vi "Main-GUI-v2.vi"() -> ()   [LabVIEW 2021]
uses:
  Controls/Command_cluster.ctl
  Controls/Command_Enum.ctl
  Controls/AR-msg-variables.ctl
  Controls/AR-com-ports.ctl
  Controls/AR-instrument-refs.ctl
  C:/Projects/Automation/nLight Laser/nlight_dll/altaAPI.dll
  Automation/nLight Laser/nlight_dll/altaAPI.dll
  Controls/AR-axis-parameters.ctl
  Automation/Zaber Stage/Controls/Zaber-parameters.ctl
  Controls/AR-Interlock-Data.ctl
  Automation/nLight Laser/Controls/CW-Laser-params.ctl
  Automation/nLight Laser/Controls/Status-flags.ctl
  Automation/nLight Laser/Controls/nLight-beam-modes.ctl
  Controls/AR-Interlock-monitor-comands.ctl
  Automation/nLight Laser/Controls/nLight-wait-states.ctl
  <instrlib>/Zaber A Series/Zaber A Series.lvlib
panel:
  in  "Stop 2":bool caption="Stop"
  in  "EMIT!":bool
  out "Accel Active":bool
  out "msg-var at exit":T1={"Run Rcp"=FALSE, "Rcp Stopped"=FALSE, "Err Device"="", "Run Axis Loop"=TRUE}
  in  "Simulate Laser":bool
  in  "Axis params":T2={"X"={"Device (dev axis)"="1 3", "Lockstep Group (1)"=1, "Units"=enum."millimeters", "Microstep Size"=4.21875, "Move (units)"=1500.0, "Direction(-1,1)"=1, "Speed (units/s)"=0.0}, "Y"={"Device (dev axis)"="1", "Lockstep Group (1)"=1, "Units"=enum."millimeters", "Microstep Size"=0.496094, "Move (units)"=0.0, "Direction(-1,1)"=1, "Speed (units/s)"=0.0}}
  in  "Tab Control":T4(tab)
  in  "Re-test gating":bool
  in  "X Axis Initial Test Parameters":T3={"Device (dev axis)"="1 3", "Lockstep Group (1)"=1, "Units"=enum."millimeters", "Microstep Size"=4.21875, "Move (units)"=1500.0, "Direction(-1,1)"=1, "Speed (units/s)"=0.0}
  out "MCU INLK":bool=TRUE
  in  "Init":bool
  out "Laser OK":bool
  in  "Com ports":T5={"Zaber Com"="COM3", "MCU Com"="COM5", "Laser IP"="172.30.0.50", "Laser Com"=""}
  in  "Recipe (csv)":path=path "C:/Projects/Alpha Redux"
  out "Zaber OK":bool=TRUE
  out "Controll Interface":i32(ring) items=["HW", "API", "CLI", "INET, CONTROL_INT_MASK"]
  out "External Gate":bool
  out "Profile Mode":bool
  out "Gating Timedout":bool
  out "X Position Triggered":dbl
  out "Delta Time (mS)":dbl
  out "MCU Gating Flags":T6
  out "error out":errorcluster
  in  "Save script":bool
  in  "Load script":bool
  in  "Script":T7[](array[typedef])=[{"Step#"=10.0, "Commands"=enum."Home All", "Parameter1"=0.0, "Parameter2"=0.0, "Parameter3"=0.0}, {"Step#"=20.0, "Commands"=enum."Y Move Rel", "Parameter1"=20.0, "Parameter2"=1.0, "Parameter3"=0.0}, {"Step#"=30.0, "Commands"=enum."Wait", "Parameter1"=500.0, "Parameter2"=0.0, "Parameter3"=0.0}, {"Step#"=40.0, "Commands"=enum."X Move Abs", "Parameter1"=300.0, "Parameter2"=0.0, "Parameter3"=0.0}, {"Step#"=50.0, "Commands"=enum."Wait", "Parameter1"=1000.0, "Parameter2"=0.0, "Parameter3"=0.0}, {"Step#"=60.0, "Commands"=enum."Y Move Rel", "Parameter1"=10.0, "Parameter2"=-1.0, "Parameter3"=0.0}, {"Step#"=70.0, "Commands"=enum."Wait", "Parameter1"=500.0, "Parameter2"=0.0, "Parameter3"=0.0}, {"Step#"=80.0, "Commands"=enum."X Move Abs", "Parameter1"=50.0, "Parameter2"=0.0, "Parameter3"=0.0}, {"Step#"=90.0, "Commands"=enum."Wait", "Parameter1"=1000.0, "Parameter2"=0.0, "Parameter3"=0.0}, {"Step#"=100.0, "Commands"=enum."Repeat", "Parameter1"=20.0, "Parameter2"=5.0, "Parameter3"=0.0}, {"Step#"=110.0, "Commands"=enum."Y Move Abs", "Parameter1"=10.0, "Parameter2"=0.0, "Parameter3"=0.0}, {"Step#"=120.0, "Commands"=enum."End", "Parameter1"=0.0, "Parameter2"=0.0, "Parameter3"=0.0}]
  in  "Y Microstep Size":dbl=0.496094
  in  "X Microstep Size":dbl=4.21875
  in  "Y (dev axis)":string="1"
  in  "X (dev axis)":string="1 3"
  in  "Select Units":T9(ring)=enum."millimeters"
  in  "Zaber settings":bool
  out "Device Info":T10(array[cluster])=[{"Motion Type"="Linear", "Device Name"="X-MCC3 (rev 2) Controller + LRQ150BL-DE51T10A", "Microstep Size"=0.49609375000198436}, {"Motion Type"="Linear", "Device Name"="X-MCC3 (rev 2) Controller + LRQ150BL-DE51T10A", "Microstep Size"=0.49609375000198436}, {"Motion Type"="Linear", "Device Name"="X-MCC3 (rev 2) Controller + BLQ2095-E01T3A", "Microstep Size"=4.2187499996625}] {"Microstep Size" format="%#_6f"}
  out "Devices":string[](array[string])=["1"]
  out "Axis":string[](array[string])=["3"]
  out "sys on":bool
  in  "Use Saved Position":bool
  out "Aiming RDY":bool
  in  "AIMING":bool
  out "Mode RDY":bool
  in  "Beam-profile(0-6)":T11
  in  "X Speed mm/s":dbl=500.0
  in  "Clear":bool
  in  "Request":bool
  out "Gating Data":T12={"Application"="", "Msg#"=0, "uS time"=0, "Gate"=TRUE, "Head"=TRUE, "Head Old"=FALSE, "Chamber Ena"=FALSE, "Profiler Ena"=FALSE, "OPower Ena"=FALSE, "Gate Ena"=FALSE, "Time Delta (mS)"=0.0, "Head F Edge"=FALSE} {"Time Delta (mS)" format="%#_3f"}
  out "MCU Gating Raw Output":string
  out "Laser Msg Log":string
  in  "Laser Params":T13={"Power(W)"=30.0, "Duty(%)"=5.0, "Freq(Hz)"=1000.0}
  in  "SysON":bool
  in  "ENA":bool
  in  "Set Laser Params":bool caption="Set"
  out "Laser Status":T14
  out "Current Y Pos":dbl
  in  "Y Home":bool
  in  "Y Abs":bool
  in  "Y Abs Units":dbl=50.0
  out "Current X Pos":dbl=-3.9234375
  in  "X Home":bool
  in  "X Abs":bool
  in  "X Abs Units":dbl=500.0
  in  "Y Units":dbl=1.0
  in  "X Units":dbl=10.0
  in  "Y Front":bool
  in  "Y Back":bool
  in  "X Left":bool
  in  "X Right":bool
  in  "Saved Positions":string[][](table)=[["Chamber", "1005", "75"], ["Power Meter", "1500", "73"], ["", "", ""]]
  out "ena":bool
  in  "Head Flag\nLenght (mm)":dbl=100.0
  in  "Run script":bool
  in  "Stop":bool
  in  "Next":bool
  in  "Step":bool
  out "Y Position":dbl
  out "X Position":dbl
  out "Gate Trigger":cluster{dbl[], i16[]}(graph) caption="XY Graph - Light"
  out "Speeds (m/s)":dbl[](array[numeric])
  out "X Axis Pos/Speed":cluster{u32[], dbl[]}(graph) caption="XY Graph - Light"
  in  "Select":bool
  out "Laser Status":T14
  out "Laser Power (W)":dbl
  out "Laser Duty (%)":dbl
  out "Next command":T7
  in  "Target Time (s)":dbl=1.0
  in  "Accel COM":refnum<visa-resource-name>
  in  "Accel CSV File":path=path "C:/Users/cleanroom/Desktop/Accelerometer Files/Test1.csv"
  in  "Accel Ena":bool caption="ENABLE"
  out "File OK":bool
  out "Com\nError":bool
  out "Instr Refs":T15={"Zaber Com"="COM21", "MCU Com"="COM22", "LaserSysRef Out"=refnum, "LaserControl Ref Out"=refnum}
  in  "error in":errorcluster
  out "msg-var":T1={"Run Rcp"=FALSE, "Rcp Stopped"=FALSE, "Err Device"="", "Run Axis Loop"=TRUE}
  in  "Quit":bool
  out "Action":string="Quit"
  # "Emit not used\nwith EXT TRIG"
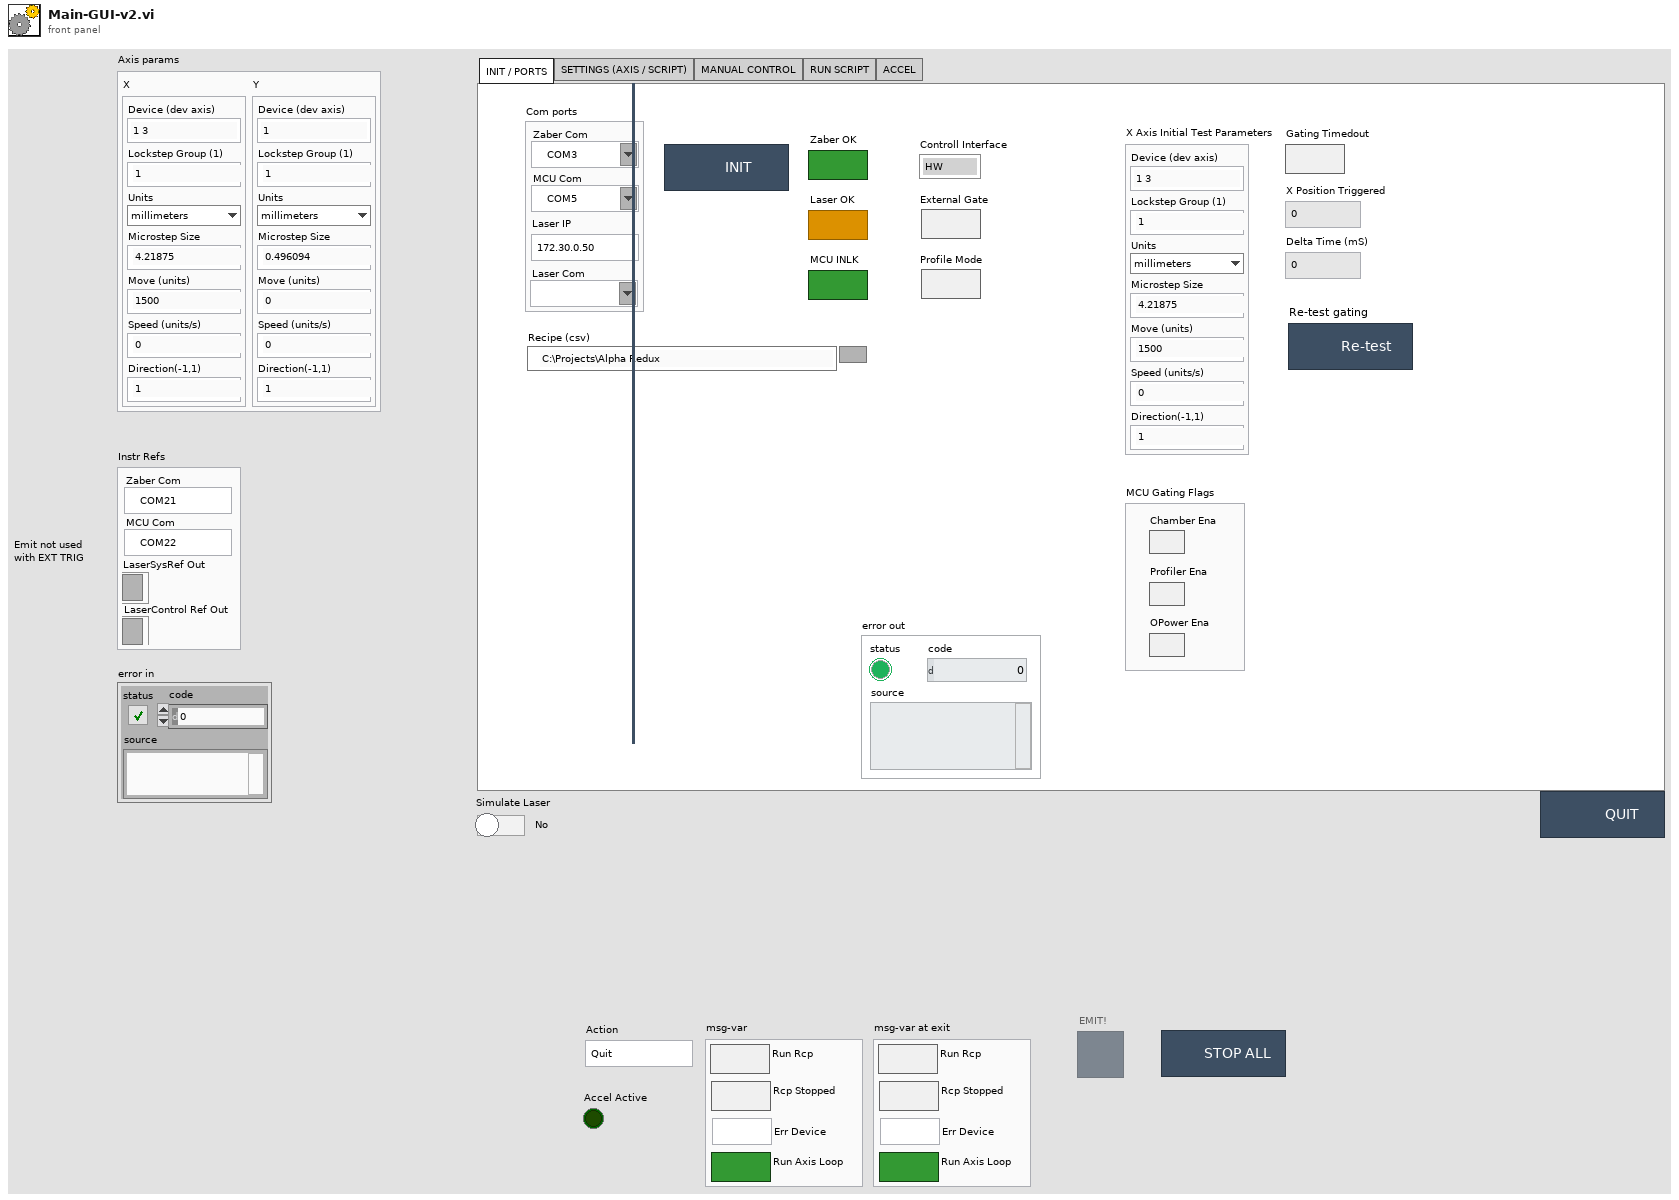
[diagram p1: front panel]
types:
  T1 = typedef "AR-msg-variables.ctl" = cluster{"Run Rcp":bool, "Rcp Stopped":bool, "Err Device":string, "Run Axis Loop":bool}
  T2 = typedef "AR-axis-parameters.ctl" = cluster{"X":T3, "Y":T3}
  T3 = typedef "Zaber-parameters.ctl" = cluster{"Device (dev axis)":string, "Lockstep Group (1)":u8, "Units":enum16{"microsteps", "microns", "millimeters", "inches", "degrees"}, "Microstep Size":dbl, "Move (units)":dbl, "Direction(-1,1)":i32, "Speed (units/s)":dbl}
  T4 = enum32{"INIT / PORTS", "SETTINGS (AXIS / SCRIPT)", "MANUAL CONTROL", "RUN SCRIPT", "ACCEL"}
  T5 = typedef "AR-com-ports.ctl" = cluster{"Zaber Com":refnum<visa-resource-name>, "MCU Com":refnum<visa-resource-name>, "Laser IP":string, "Laser Com":refnum<visa-resource-name>}
  T6 = cluster{"Chamber Ena":bool, "Profiler Ena":bool, "OPower Ena":bool}
  T7 = typedef "Command_cluster.ctl" = cluster{"Step#":dbl, "Commands":T8, "Parameter1":dbl, "Parameter2":dbl, "Parameter3":dbl}
  T8 = typedef "Command_Enum.ctl" = enum16{"End", "Home All", "X Home", "Y Home", "X Move Rel", "X Move Abs", "Y Move Rel", "Y Move Abs", "Wait", "Repeat", "Reset Intlk Timer", "Laser Sys ON", "Laser ENA"}
  T9 = enum16{"microsteps", "microns", "millimeters", "inches", "degrees"}
  T10 = cluster{"Motion Type":string, "Device Name":string, "Microstep Size":dbl}[]
  T11 = typedef "nLight-beam-modes.ctl" = enum32{"0/100 single-mode", "30/70", "40/60", "50/50", "60/40", "80/20", "90/10 max donut"}
  T12 = typedef "AR-Interlock-Data.ctl" = cluster{"Application":string, "Msg#":i32, "uS time":u32, "Gate":bool, "Head":bool, "Head Old":bool, "Chamber Ena":bool, "Profiler Ena":bool, "OPower Ena":bool, "Gate Ena":bool, "Time Delta (mS)":dbl, "Head F Edge":bool}
  T13 = typedef "CW-Laser-params.ctl" = cluster{"Power(W)":dbl, "Duty(%)":dbl, "Freq(Hz)":dbl}
  T14 = typedef "Status-flags.ctl" = cluster{"SystemOn":bool, "Enabled":bool, "LaserOn":bool, "Standby":bool, "Interlock":bool, "Error":bool, "Warning":bool, "Fault":bool}
  T15 = typedef "AR-instrument-refs.ctl" = cluster{"Zaber Com":refnum<visa-resource-name>, "MCU Com":refnum<visa-resource-name>, "LaserSysRef Out":refnum<k24>, "LaserControl Ref Out":refnum<k24>}
  T16 = enum32{"INIT / PORTS", "SETTINGS (AXIS / SCRIPT)", "MANUAL CONTROL", "RUN SCRIPT"}
  T17 = enum32{"Page Enabled", "Page Disabled", "Page Disabled & Grayed"}
  T18 = typedef "AR-Interlock-monitor-comands.ctl" = enum16{"Init", "Request", "Poll Serial", "Close", "Clear Data"}
  T19 = typedef "LVRowAndColumnTypeDef.ctl" = cluster{"Row":i32, "Column":i32}
  T20 = enum8{"Enabled", "Disabled", "Disabled and Grayed Out"}
  T21 = typedef "nLight-wait-states.ctl" = enum16{"Wait SysON", "Wait ENA", "Wait SysOFF", "Wait DIS", "No Wait"}
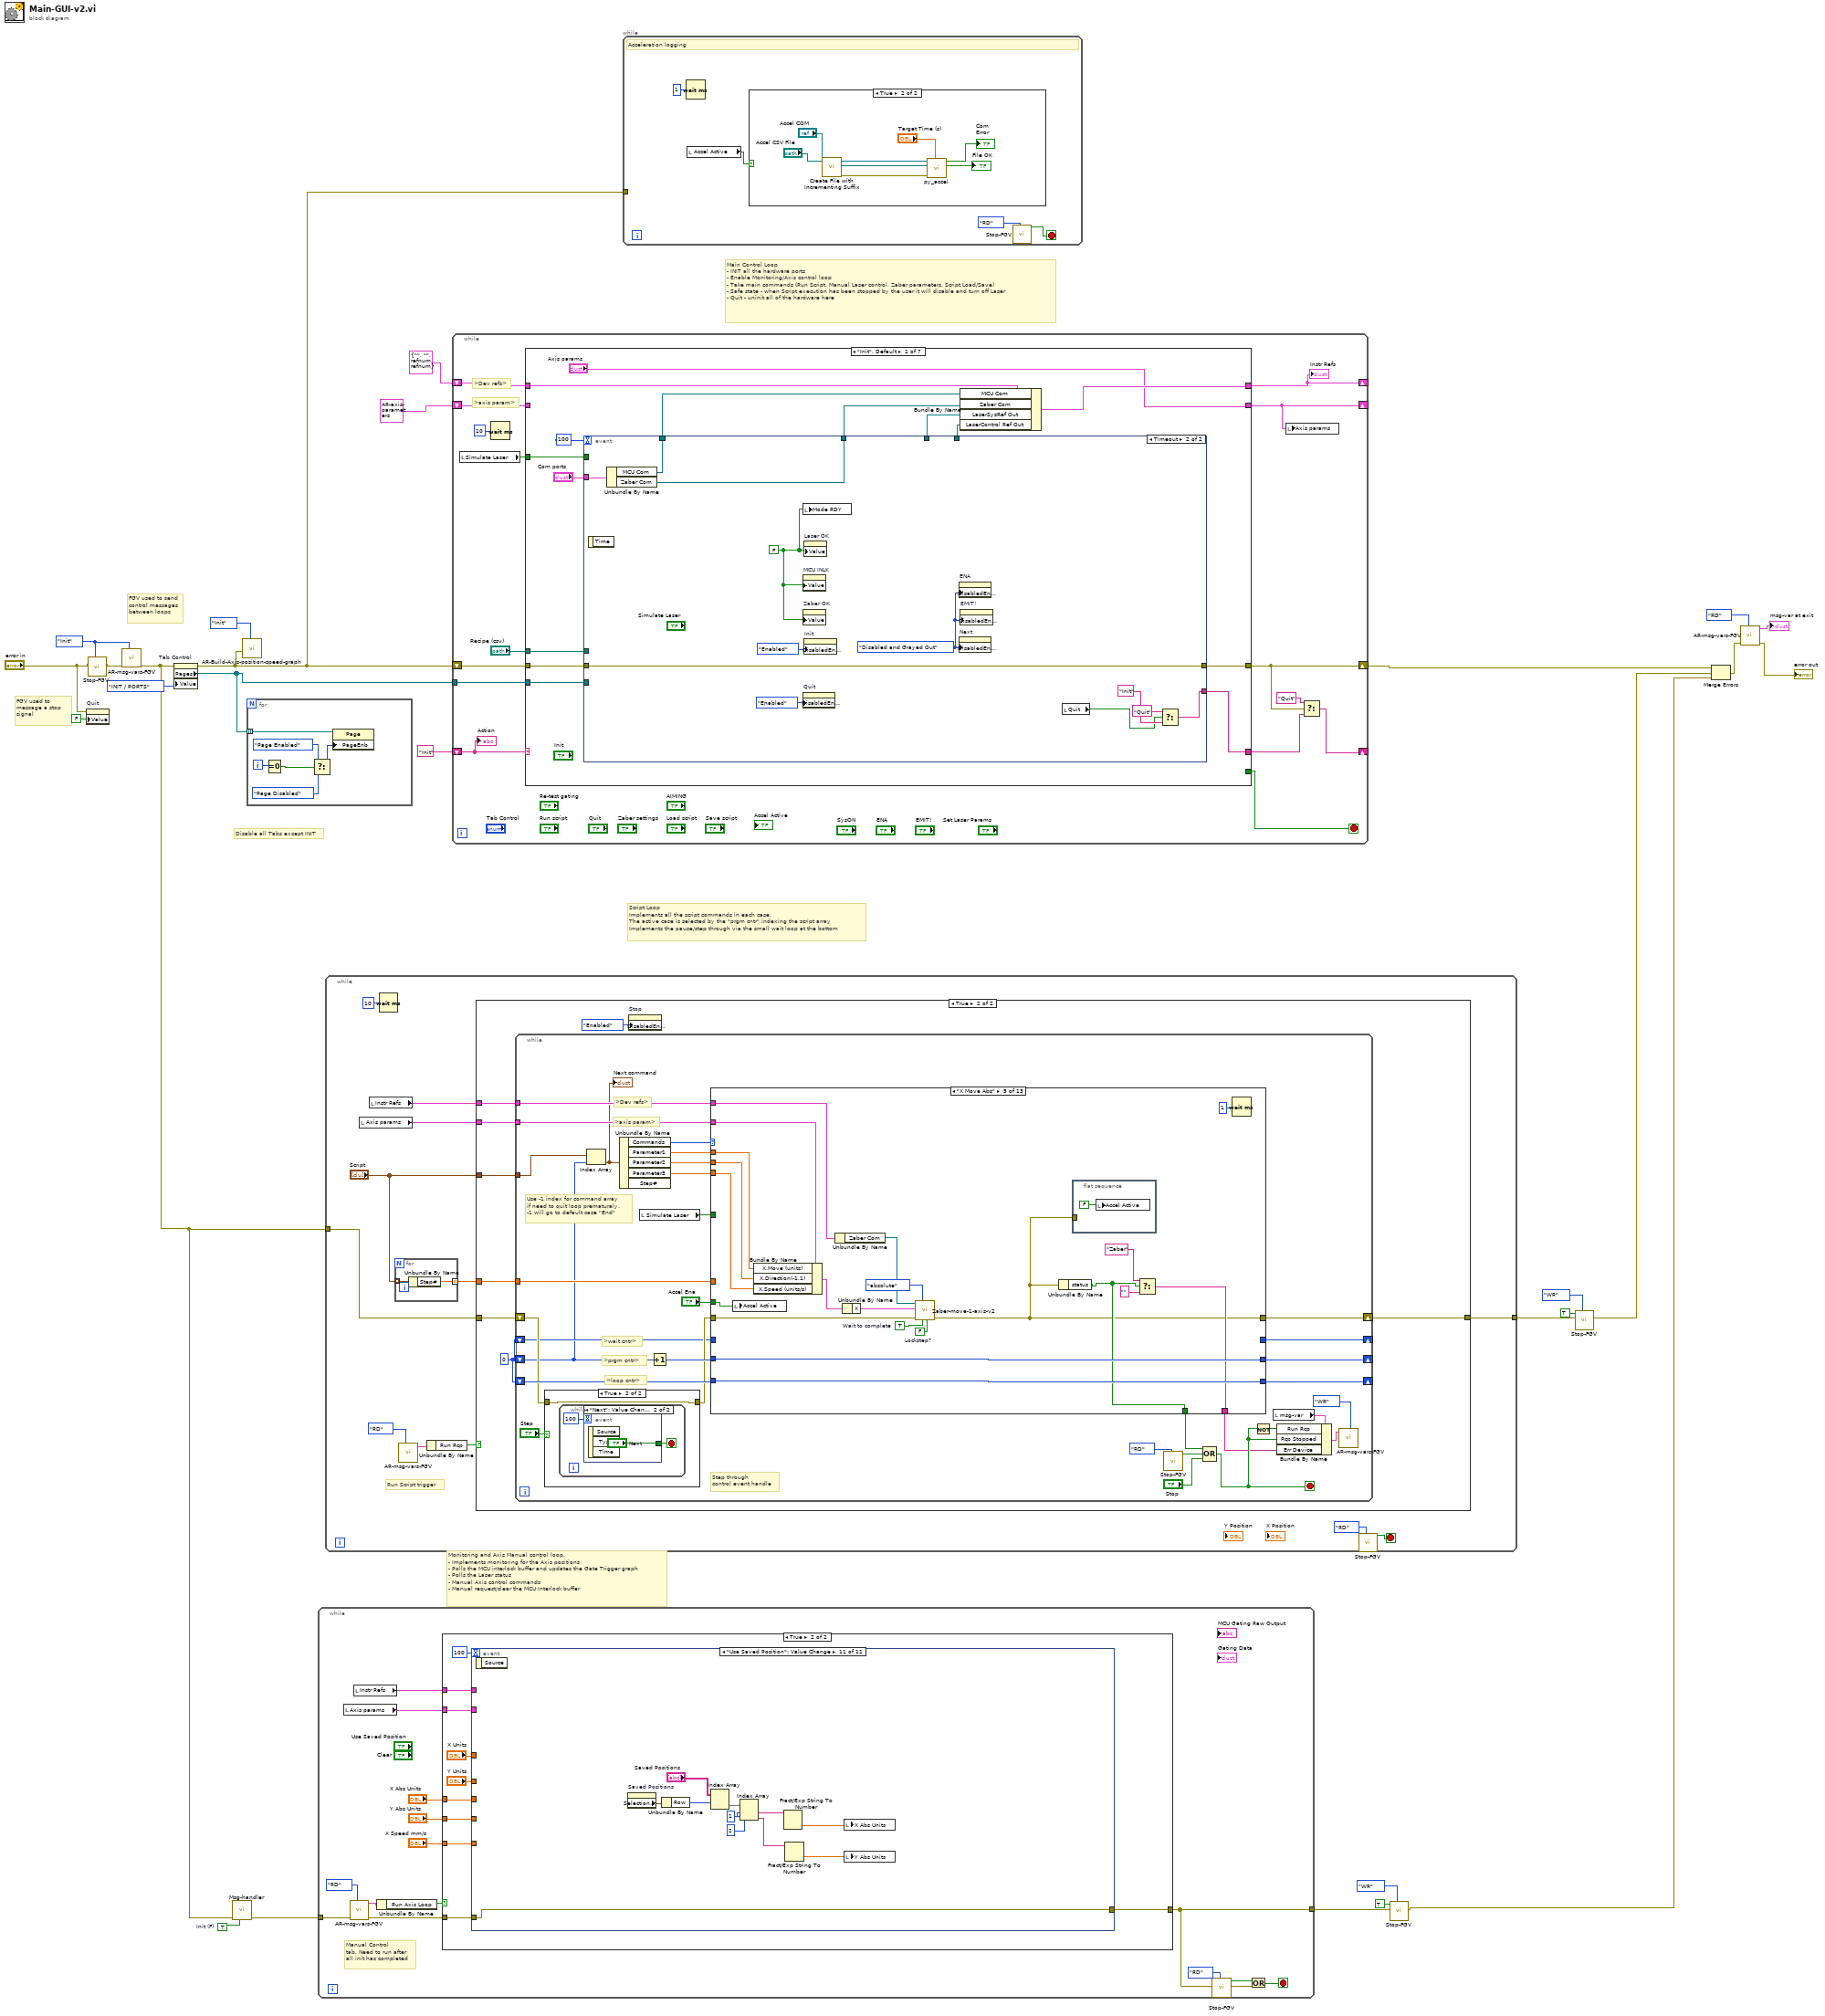
[diagram p0: block diagram]
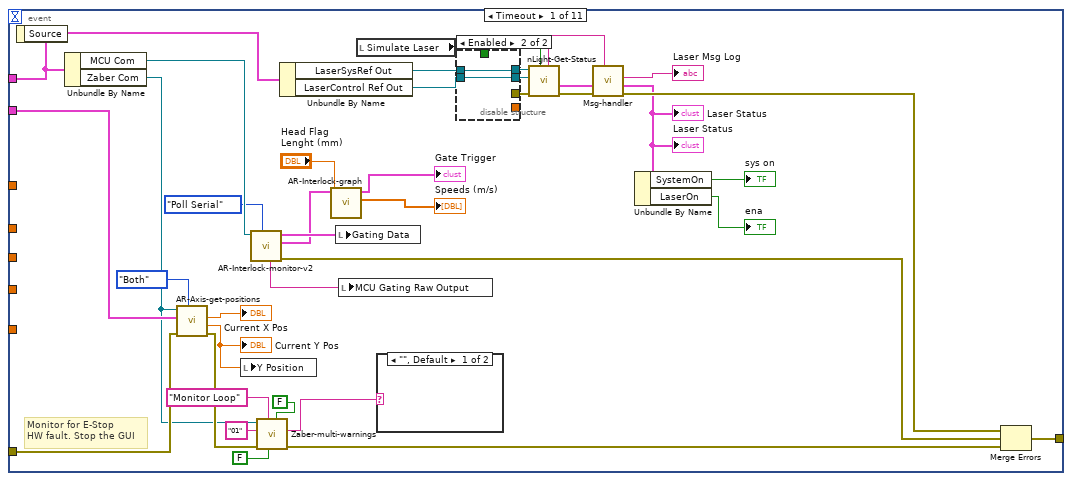
[diagram p4: hidden frame]
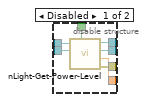
[diagram p5: hidden frame]
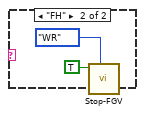
[diagram p6: hidden frame]
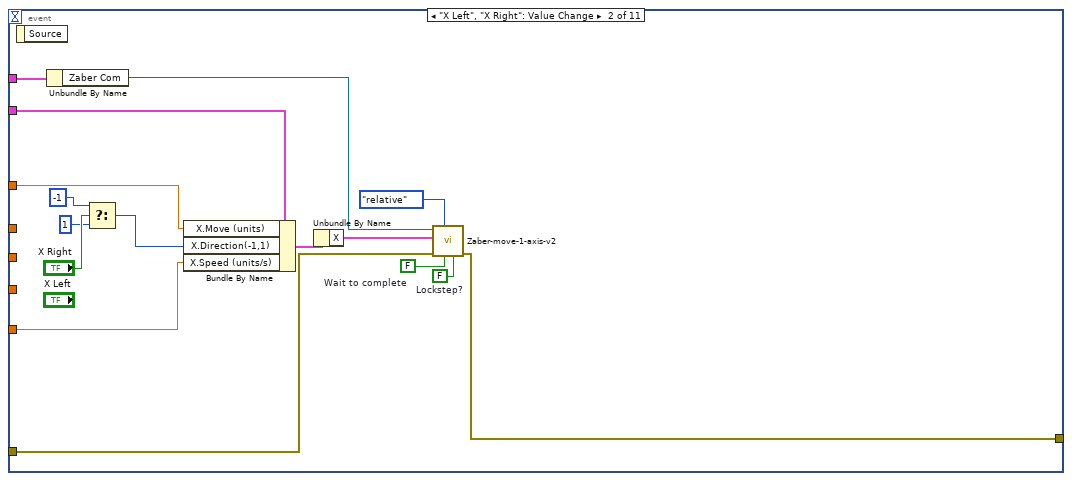
[diagram p7: hidden frame]
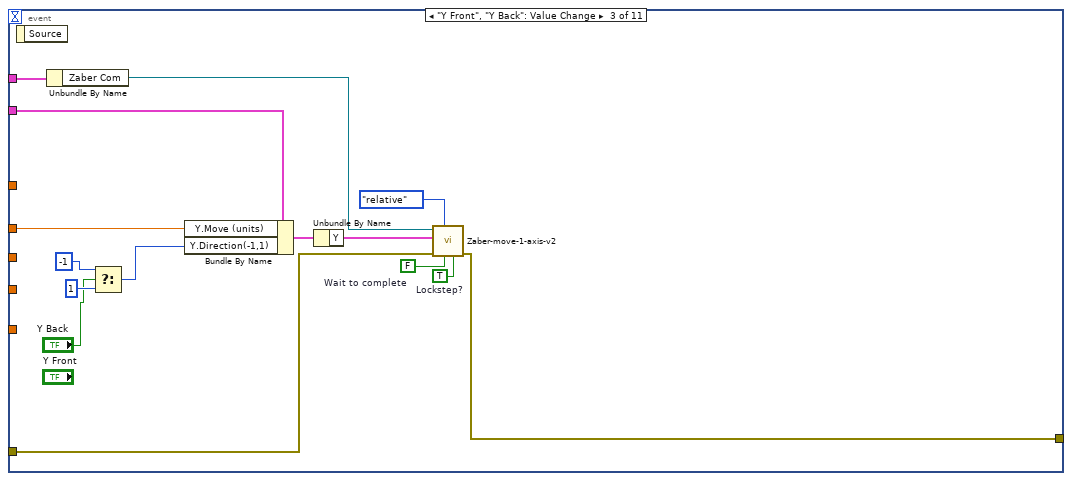
[diagram p8: hidden frame]
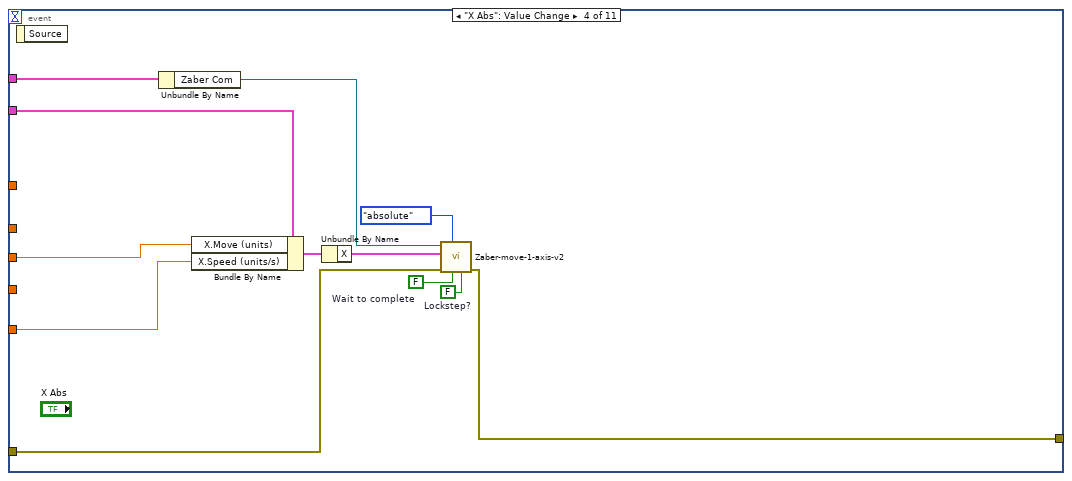
[diagram p9: hidden frame]
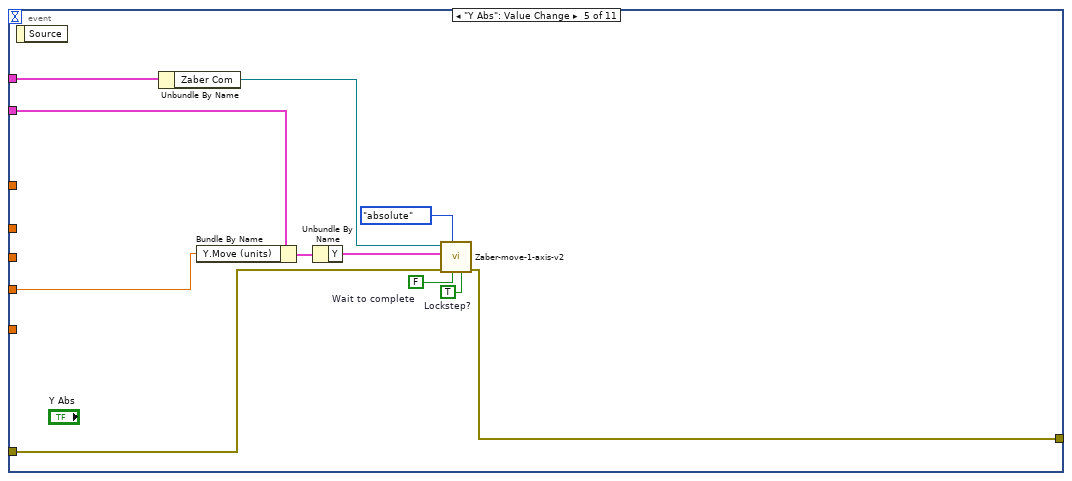
[diagram p10: hidden frame]
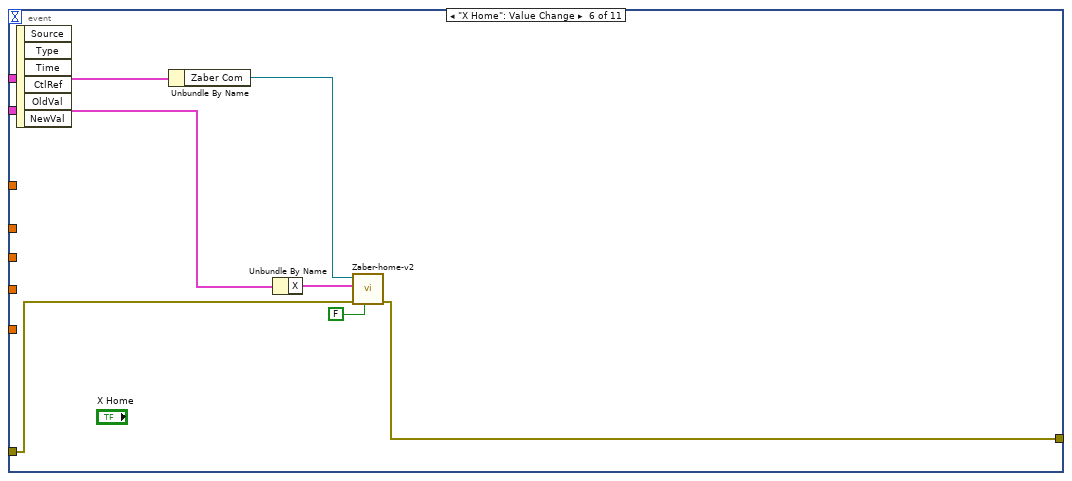
[diagram p11: hidden frame]
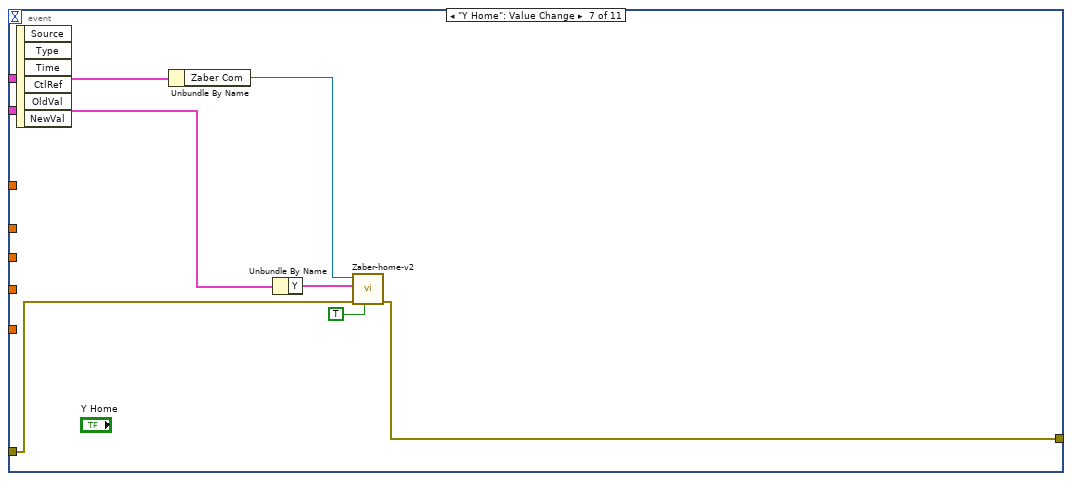
[diagram p12: hidden frame]
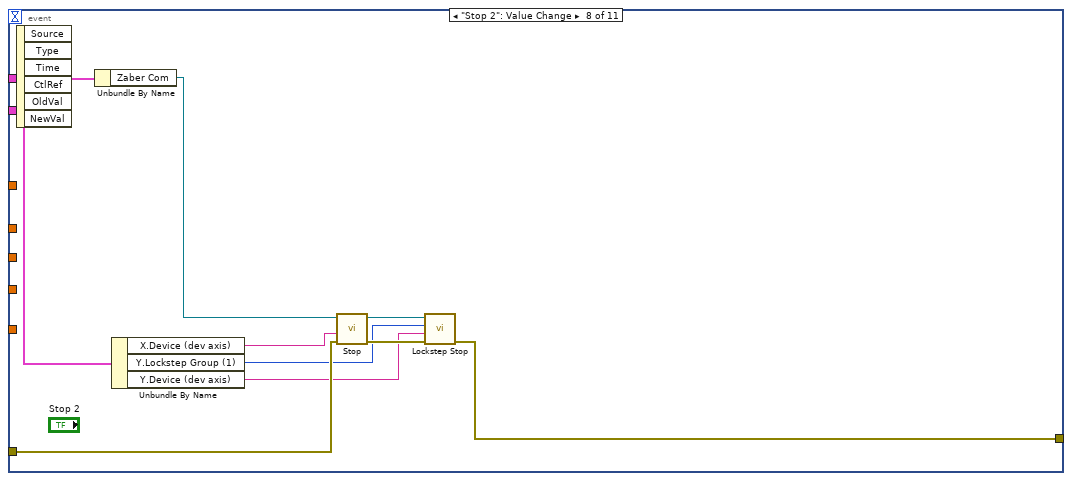
[diagram p13: hidden frame]
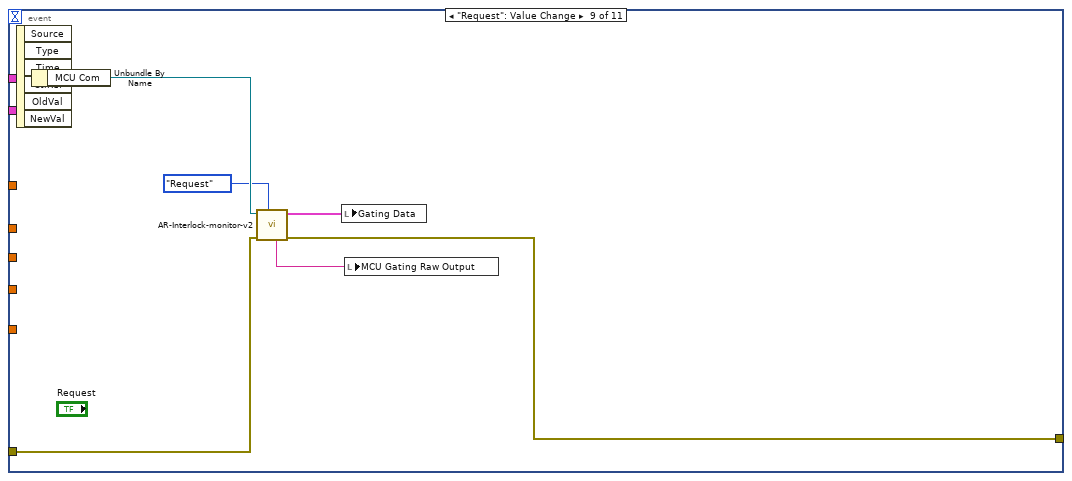
[diagram p14: hidden frame]
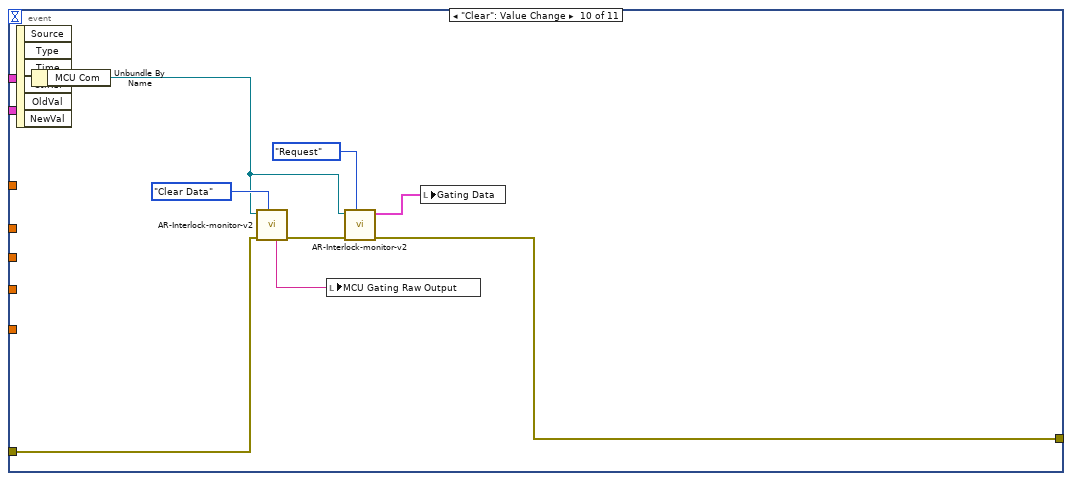
[diagram p15: hidden frame]
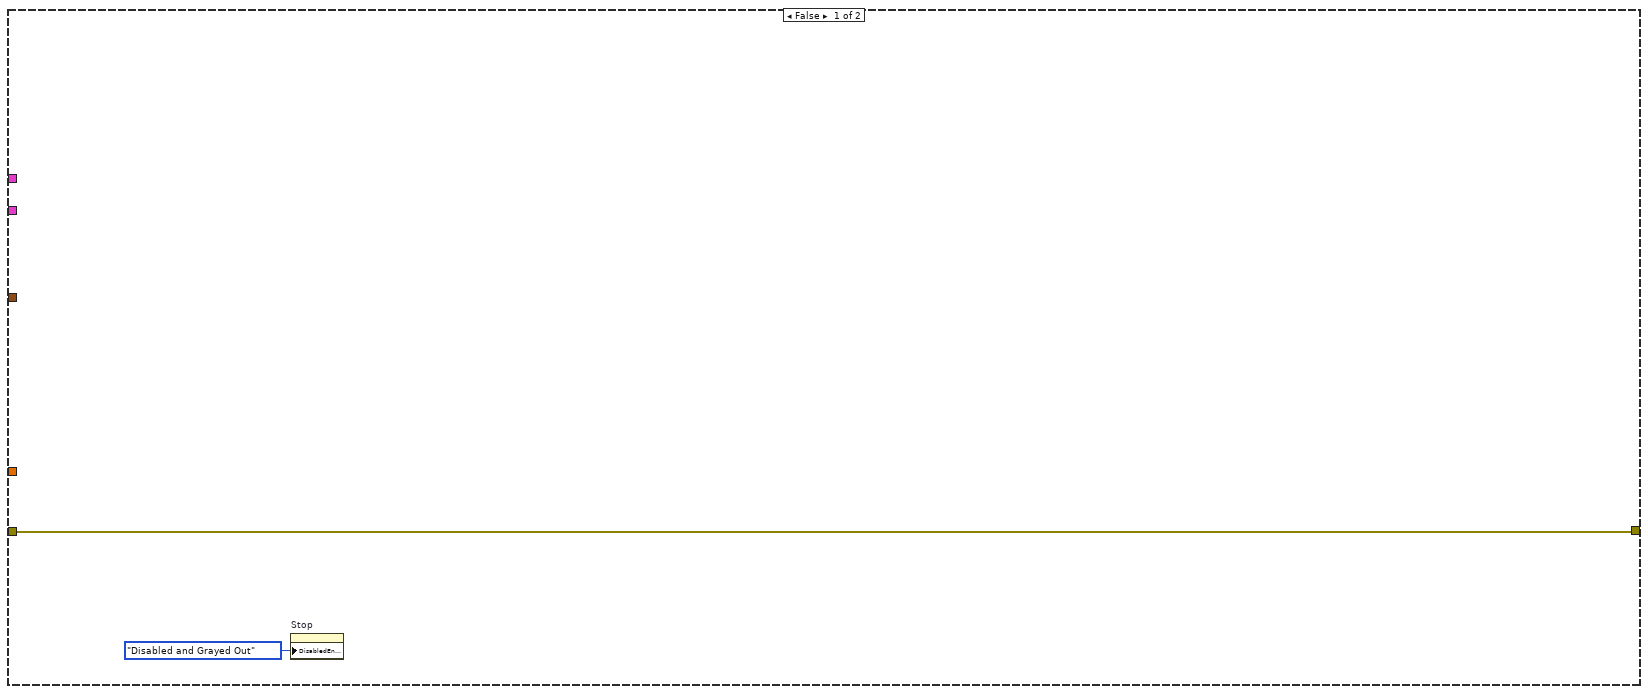
[diagram p16: hidden frame]
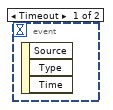
[diagram p18: hidden frame]
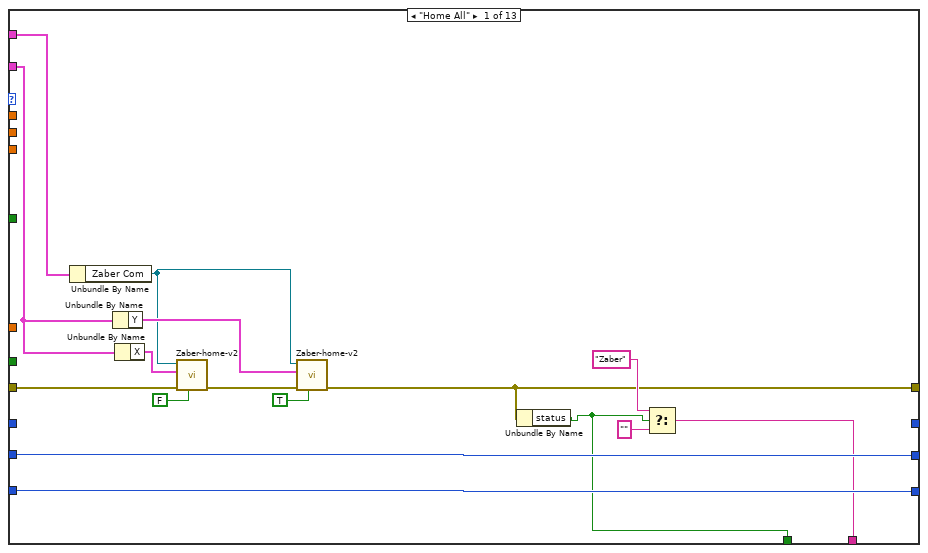
[diagram p19: hidden frame]
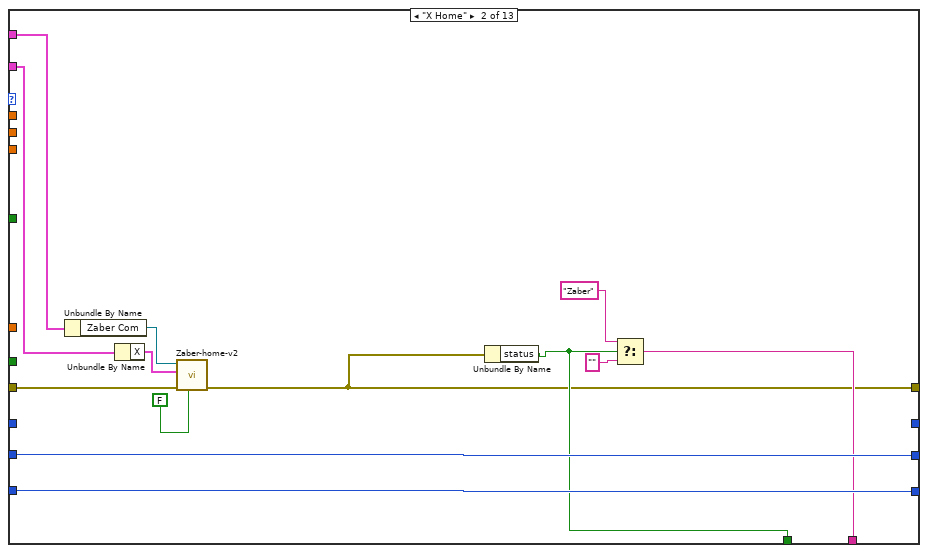
[diagram p20: hidden frame]
diagram:
  w19 = TRUE  # Init (F)
  w25 = enum16{"Init", "WR", "RD"}."Init" ("Action (RD)")
  # "Monitoring and Axis Manual control loop.\n- Implements monitoring for the Axis positions\n- Polls the MCU interlock buffer and updates the Gate Trigger graph\n- Polls the Laser status\n- Manual Axis control commands\n- Manual request/clear the MCU Interlock buffer"
  # "Main Control Loop\n- INIT all the hardware ports \n- Enable Monitoring/Axis control loop\n- Take main commands (Run Script, Manual Laser control, Zaber parameters, Script Load/Save)\n- Safe state - when Script execution has been stopped by the user it will disable and turn off Laser\n- Quit - uninit all of the hardware here"
  # "Disable all Tabs except INIT"
  # "FGV used to send control messages between loops"
  # "FGV used to \nmessage a stop\nsignal"
  # "Script Loop\nImplements all the script commands in each case.\nThe active case is selected by the \"prgm cntr\" indexing the script array\nImplements the pause/step through via the small wait loop at the bottom"
  n1 = property on="Quit" class="Bool (strict)"(error in="error in", "Value"=FALSE ("Quit")) -> ()  [unwired: 1 in, 2 out]
  n2 = call "Stop-FGV.vi"("Action (RD)"=w25, "error in"="error in") -> ("error out"=w26:errorcluster)  [unwired: 8 in, 1 out]
  n3 = call "AR-msg-vars-FGV.vi"("Action"=w25, "error in"=w26) -> ("error out"=w18:errorcluster)  [unwired: 8 in, 1 out]
  n4 = property on="Tab Control" class="TabCtl (strict)"(error in=w18, "Value"=T16."INIT / PORTS" ("Tab Control")) -> (error out=w3:errorcluster, "Pages"=w22:refnum<vi>[])  [unwired: 1 in, 1 out]
  n5 = call "Msg-handler.vi"("Init (F)"=w19, "error in"=w18) -> ("error out"=w17:errorcluster)  [unwired: 6 in, 3 out]
  n6 = call "AR-Build-Axis-position-speed-graph.vi"("Action"=enum16{"Init", "WR", "RD"}."Init", "error in (no error)"=w3) -> ()  [unwired: 9 in, 1 out]
  n7 = for {
    tunnel: w22 -> [w33] mode=indexing
    i -> [w32]
    n8 = Equal To 0?(x=w32) -> (x = 0?=w31:bool)
    n9 = Select(t=T17."Page Enabled" ("Page Enabled State"), s=w31, f=T17."Page Disabled" ("Page Enabled State")) -> (s? t:f=w28:T17)
    n10 = property class="Page"(reference=w33, "PageEnb"=w28) -> ()  [unwired: 1 in, 2 out]
  }
  n11 = while {
    tunnel: w17 -> [w42]
    tunnel: [w36] -> w11
    stop <- w40 stop-if-true
    # "Manual Control\ntab. Need to run after\nall init has completed"
    n12 = local read "Axis params"() -> (w43:T2)
    n13 = call "AR-msg-vars-FGV.vi"("Action"=enum16{"Init", "WR", "RD"}."RD", "error in"=w42) -> ("error out"=w41:errorcluster, "msg-var"=w47:T1)  [unwired: 8 in]
    n14 = local read "Instr Refs"() -> (w44:T15)
    n15 = Unbundle By Name(w47) -> ("Run Axis Loop"=w45:bool)
    n16 = case shown="True" w45 {
      tunnel: w44 -> [_ w59]
      tunnel: w43 -> [_ w58]
      tunnel: w41 -> [w49 w57]
      tunnel: [w49 w56] -> w36
      tunnel: "X Abs Units" -> [_ w52]
      tunnel: "Y Abs Units" -> [_ w51]
      tunnel: "X Speed mm/s" -> [_ w50]
      frame False {
      }
      frame True {
        # "Run Sequence"
        n17 = event shown="[10] \"Use Saved Position\": Value Change" {
          selector: _ -> [_ _ _ _ _ _ _ _ _ _ _]
          dyn-events: _ -> [_ _ _ _ _ _ _ _ _ _ _]
          timeout: 100 -> [_ _ _ _ _ _ _ _ _ _ _]
          tunnel: w59 -> [w80 w114 w130 w145 w156 w166 w173 w186 w189 w201 _]
          tunnel: w58 -> [w96 w115 w131 w146 w157 w165 w172 w180 _ _ _]
          tunnel: w57 -> [w95 w112 w128 w142 w154 w164 w171 w183 w191 w202 w213]
          tunnel: [w90 w111 w127 w141 w153 w163 w170 w181 w190 w198 w213] -> w56
          tunnel: "Y Units" -> [_ _ w125 _ _ _ _ _ _ _ _]
          tunnel: "X Units" -> [_ w110 _ _ _ _ _ _ _ _ _]
          tunnel: w52 -> [_ _ _ w143 _ _ _ _ _ _ _]
          tunnel: w51 -> [_ _ _ _ w152 _ _ _ _ _ _]
          tunnel: w50 -> [_ w109 _ w140 _ _ _ _ _ _ _]
          event Timeout {
            # "Monitor for E-Stop\nHW fault. Stop the GUI"
            n18 = event-data() -> ()  [unwired: 1 in, 1 out]
            n19 = Unbundle By Name(w80) -> ("MCU Com"=w93:refnum<visa-resource-name>, "Zaber Com"=w69:refnum<visa-resource-name>)
            n20 = call "AR-Axis-get-positions.vi"("Select"=enum16{"X Axis", "Y Axis", "Both"}."Both", "error in"=w95, "Axis params"=w96, "Port In"=w69) -> ("error out"=w70:errorcluster, "Y Pos"=w84:dbl, "X Pos"=→"Current X Pos":dbl)  [unwired: 4 in, 1 out]
            "Current Y Pos" <- w84
            n21 = local write "Y Position"(w84) -> ()
            n22 = call "AR-Interlock-monitor-v2.vi"("Action"=AR-Interlock-monitor-comands."Poll Serial", "Inlk Com"=w93) -> ("error out"=w91:errorcluster, "Intlk Data Array"=w87:T12[], "Intlk Data"=w88:T12, "Raw Output"=w89:string)  [unwired: 5 in, 1 out]
            n23 = call "Zaber-multi-warnings.vi"("Log?"=FALSE, "Msg?"=FALSE, "LogSource"="Monitor Loop", "error in"=w70, "Device"="01", "Com Port"=w69) -> ("error out"=w65:errorcluster, "Warning Flag"=w64:string)  [unwired: 2 in, 2 out]
            n24 = Unbundle By Name(w80) -> ("LaserSysRef Out"=w77:refnum<k24>, "LaserControl Ref Out"=w75:refnum<k24>)
            n25 = call "AR-Interlock-graph.vi"("Flag Lenght (mm)"="Head Flag\nLenght (mm)", "Intlk Data Array"=w87) -> ("Speeds (m/s)"=→"Speeds (m/s)":dbl[], "Gate"=→"Gate Trigger":cluster{dbl[], i16[]})  [unwired: 7 in, 1 out]
            n26 = local write "Gating Data"(w88) -> ()
            n27 = local write "MCU Gating Raw Output"(w89) -> ()
            n28 = local read "Simulate Laser"() -> (w72:bool)
            n29 = case shown="\"\", Default" w64 {
              frame "", Default {
              }
              frame "FH" {
                n30 = call "Stop-FGV.vi"("Action (RD)"=enum16{"Init", "WR", "RD"}."WR", "Action"=TRUE) -> ()  [unwired: 8 in, 2 out]
              }
            }
            n31 = disable-structure shown="Enabled" {
              disable-tunnel: w77 -> [w104 w105]
              disable-tunnel: [w103 w105] -> w76
              disable-tunnel: w75 -> [w102 w106]
              disable-tunnel: [w101 w106] -> w74
              disable-tunnel: [w100 _] -> w73
              disable-tunnel: [w99 _] -> _
              disable-tunnel: w72 -> [w98 _]
              frame Disabled {
                n32 = call "nLight-Get-Power-Level.vi"("Simulate (F)"=w98, "LaserControl Ref"=w102, "LaserSysRef"=w104) -> ("error out"=w100:errorcluster, "PowerOutput"=w99:dbl, "LaserControl Ref Out"=w101:refnum<k24>, "LaserSysRef Out"=w103:refnum<k24>)  [unwired: 5 in]
              }
              frame Enabled {
              }
            }
            n33 = call "nLight-Get-Status.vi"("Simulate (F)"=w72, "error in"=w73, "LaserControl Ref"=w74, "LaserSysRef"=w76) -> ("error out"=w81:errorcluster, "Status-flags"=w82:T14, "Msg"=w83:string)  [unwired: 2 in, 3 out]
            n34 = call "Msg-handler.vi"("Msg"=w83, "error in"=w81, "Status-flags"=w82) -> ("error out"=w78:errorcluster, "Status-flags Out"=w62:T14, "Msg log"=→"Laser Msg Log":string)  [unwired: 5 in, 1 out]
            "Laser Status" <- w62
            "Laser Status" <- w62
            n35 = Unbundle By Name(w62) -> ("SystemOn"=→"sys on":bool, "LaserOn"=→"ena":bool)
            n36 = Merge Errors(w78, w91, w65) -> (w90:errorcluster)
          }
          event "X Left", "X Right": Value Change {
            w119 = FALSE  # Wait to complete
            w120 = FALSE  # Lockstep?
            n37 = event-data() -> ()  [unwired: 1 in, 1 out]
            n38 = Unbundle By Name(w114) -> ("Zaber Com"=w113:refnum<visa-resource-name>)
            n39 = Select(t=-1 ("Direction(-1,1)"), s="X Right", f=1) -> (s? t:f=w123:i32)
            n40 = Bundle By Name(cluster=w115, "X.Move (units)"=w110, "X.Direction(-1,1)"=w123, "X.Speed (units/s)"=w109) -> (w116:T2)
            n41 = Unbundle By Name(w116) -> ("X"=w117:T3)
            n42 = call "Zaber-move-1-axis-v2.vi"("Lockstep?"=w120, "Wait to complete"=w119, "Movement Type"=enum16{"relative", "absolute"}."relative", "error in"=w112, "Zaber parameters"=w117, "Port In"=w113) -> ("error out"=w111:errorcluster)  [unwired: 3 in, 2 out]
          }
          event "Y Front", "Y Back": Value Change {
            w135 = FALSE  # Wait to complete
            w136 = TRUE  # Lockstep?
            n43 = event-data() -> ()  [unwired: 1 in, 1 out]
            n44 = Unbundle By Name(w130) -> ("Zaber Com"=w129:refnum<visa-resource-name>)
            n45 = Select(t=-1 ("Direction(-1,1)"), s="Y Back", f=1) -> (s? t:f=w139:i32)
            n46 = Bundle By Name(cluster=w131, "Y.Move (units)"=w125, "Y.Direction(-1,1)"=w139) -> (w132:T2)
            n47 = Unbundle By Name(w132) -> ("Y"=w133:T3)
            n48 = call "Zaber-move-1-axis-v2.vi"("Lockstep?"=w136, "Wait to complete"=w135, "Movement Type"=enum16{"relative", "absolute"}."relative", "error in"=w128, "Zaber parameters"=w133, "Port In"=w129) -> ("error out"=w127:errorcluster)  [unwired: 3 in, 2 out]
          }
          event "X Abs": Value Change {
            w150 = FALSE  # Wait to complete
            w151 = FALSE  # Lockstep?
            n49 = event-data() -> ()  [unwired: 1 in, 1 out]
            n50 = Unbundle By Name(w145) -> ("Zaber Com"=w144:refnum<visa-resource-name>)
            n51 = Bundle By Name(cluster=w146, "X.Move (units)"=w143, "X.Speed (units/s)"=w140) -> (w147:T2)
            n52 = Unbundle By Name(w147) -> ("X"=w148:T3)
            n53 = call "Zaber-move-1-axis-v2.vi"("Lockstep?"=w151, "Wait to complete"=w150, "Movement Type"=enum16{"relative", "absolute"}."absolute", "error in"=w142, "Zaber parameters"=w148, "Port In"=w144) -> ("error out"=w141:errorcluster)  [unwired: 3 in, 2 out]
          }
          event "Y Abs": Value Change {
            w161 = FALSE  # Wait to complete
            w162 = TRUE  # Lockstep?
            n54 = event-data() -> ()  [unwired: 1 in, 1 out]
            n55 = Unbundle By Name(w156) -> ("Zaber Com"=w155:refnum<visa-resource-name>)
            n56 = Bundle By Name(cluster=w157, "Y.Move (units)"=w152) -> (w158:T2)
            n57 = Unbundle By Name(w158) -> ("Y"=w159:T3)
            n58 = call "Zaber-move-1-axis-v2.vi"("Lockstep?"=w162, "Wait to complete"=w161, "Movement Type"=enum16{"relative", "absolute"}."absolute", "error in"=w154, "Zaber parameters"=w159, "Port In"=w155) -> ("error out"=w153:errorcluster)  [unwired: 3 in, 2 out]
          }
          event "X Home": Value Change {
            n59 = event-data() -> ()  [unwired: 1 in, 6 out]
            n60 = Unbundle By Name(w166) -> ("Zaber Com"=w167:refnum<visa-resource-name>)
            n61 = Unbundle By Name(w165) -> ("X"=w168:T3)
            n62 = call "Zaber-home-v2.vi"("Lockstep?"=FALSE, "error in"=w164, "Zaber parameters"=w168, "Com Port"=w167) -> ("error out"=w163:errorcluster)  [unwired: 5 in, 2 out]
          }
          event "Y Home": Value Change {
            n63 = event-data() -> ()  [unwired: 1 in, 6 out]
            n64 = Unbundle By Name(w173) -> ("Zaber Com"=w174:refnum<visa-resource-name>)
            n65 = Unbundle By Name(w172) -> ("Y"=w175:T3)
            n66 = call "Zaber-home-v2.vi"("Lockstep?"=TRUE, "error in"=w171, "Zaber parameters"=w175, "Com Port"=w174) -> ("error out"=w170:errorcluster)  [unwired: 5 in, 2 out]
          }
          event "Stop 2": Value Change {
            n67 = event-data() -> ()  [unwired: 1 in, 6 out]
            n68 = Unbundle By Name(w186) -> ("Zaber Com"=w185:refnum<visa-resource-name>)
            n69 = Unbundle By Name(w180) -> ("X.Device (dev axis)"=w179:string, "Y.Lockstep Group (1)"=w178:u8, "Y.Device (dev axis)"=w177:string)
            n70 = call <instrlib>:"Stop.vi"("error in (no error)"=w183, "Device and Axis"=w179, "VISA resource name"=w185) -> ("error out"=w182:errorcluster, "VISA resource name out"=w184:refnum<visa-resource-name>)  [unwired: 7 in]
            n71 = call <instrlib>:"Lockstep Stop.vi"("error in (no error)"=w182, "Device Number"=w177, "Lockstep Group (1)"=w178, "VISA resource name"=w184) -> ("error out"=w181:errorcluster)  [unwired: 6 in, 1 out]
          }
          event "Request": Value Change {
            n72 = event-data() -> ()  [unwired: 1 in, 6 out]
            n73 = Unbundle By Name(w189) -> ("MCU Com"=w188:refnum<visa-resource-name>)
            n74 = call "AR-Interlock-monitor-v2.vi"("Action"=AR-Interlock-monitor-comands."Request", "error in"=w191, "Inlk Com"=w188) -> ("error out"=w190:errorcluster, "Intlk Data"=w192:T12, "Raw Output"=w193:string)  [unwired: 4 in, 2 out]
            n75 = local write "Gating Data"(w192) -> ()
            n76 = local write "MCU Gating Raw Output"(w193) -> ()
          }
          event "Clear": Value Change {
            n77 = event-data() -> ()  [unwired: 1 in, 6 out]
            n78 = Unbundle By Name(w201) -> ("MCU Com"=w197:refnum<visa-resource-name>)
            n79 = call "AR-Interlock-monitor-v2.vi"("Action"=AR-Interlock-monitor-comands."Clear Data" ("t"), "error in"=w202, "Inlk Com"=w197) -> ("error out"=w199:errorcluster, "Raw Output"=w194:string)  [unwired: 4 in, 3 out]
            n80 = local write "MCU Gating Raw Output"(w194) -> ()
            n81 = call "AR-Interlock-monitor-v2.vi"("Action"=AR-Interlock-monitor-comands."Request", "error in"=w199, "Inlk Com"=w197) -> ("error out"=w198:errorcluster, "Intlk Data"=w195:T12)  [unwired: 4 in, 3 out]
            n82 = local write "Gating Data"(w195) -> ()
          }
          event "Use Saved Position": Value Change {
            n83 = event-data() -> ()  [unwired: 1 in, 1 out]
            n84 = property on="Saved Positions" class="Tbl (strict)"() -> ("Selection Start"=w212:T19)  [unwired: 2 in, 2 out]
            n85 = Unbundle By Name(w212) -> ("Row"=w211:i32)
            n86 = Index Array(array="Saved Positions", index (row)=w211) -> (element=w209:string[])  [unwired: 1 in]
            n87 = Index Array(array=w209, index #1=1 ("index"), index #2=2 ("index")) -> (element #1=w206:string, element #2=w204:string)
            n88 = Fract/Exp String To Number(string=w206) -> (number=w205:dbl)  [unwired: 3 in, 1 out]
            n89 = Fract/Exp String To Number(string=w204) -> (number=w203:dbl)  [unwired: 3 in, 1 out]
            n90 = local write "X Abs Units"(w205) -> ()
            n91 = local write "Y Abs Units"(w203) -> ()
          }
        }
      }
    }
    n92 = call "Stop-FGV.vi"("Action (RD)"=enum16{"Init", "WR", "RD"}."RD", "error in"=w36) -> ("error out"=w34:errorcluster, "Out"=w35:bool)  [unwired: 8 in]
    n93 = Or(x=w35, y=w34) -> (x .or. y?=w40:bool)
  }
  n94 = while {
    tunnel: w18 -> [w222]
    tunnel: [w214] -> w16
    stop <- w225 stop-if-true
    # "Run Script trigger"
    n95 = local read "Axis params"() -> (w218:T2)
    n96 = local read "Instr Refs"() -> (w219:T15)
    n97 = Wait (ms)(milliseconds to wait=u32 10) -> ()  [unwired: 1 out]
    n98 = for {
      tunnel: "Script" -> [w529] mode=indexing
      tunnel: [w528] -> w217 mode=indexing
      n99 = Unbundle By Name(w529) -> ("Step#"=w528:dbl)
    }
    n100 = call "AR-msg-vars-FGV.vi"("Action"=enum16{"Init", "WR", "RD"}."RD") -> ("msg-var"=w221:T1)  [unwired: 9 in, 1 out]
    n101 = Unbundle By Name(w221) -> ("Run Rcp"=w216:bool)
    n102 = case shown="True" w216 {
      tunnel: w217 -> [_ w235]
      tunnel: "Script" -> [_ w234]
      tunnel: w222 -> [w227 w233]
      tunnel: w219 -> [_ w232]
      tunnel: w218 -> [_ w231]
      tunnel: [w227 w230] -> w214
      frame False {
        n103 = property on="Stop" class="Bool"("DisabledEnum"=T20."Disabled and Grayed Out" ("Disabled")) -> ()  [unwired: 2 in, 2 out]
      }
      frame True {
        w229 = 0
        # "Run Sequence"
        n104 = while {
          tunnel: w234 -> [w239]
          tunnel: w235 -> [w266]
          shift-right: [w264] -> _
          shift-left: w229 -> [w240]
          shift-right: [w261] -> _
          shift-left: w229 -> [w265]
          tunnel: w232 -> [w246]
          tunnel: w231 -> [w253]
          shift-right: [w251] -> w230
          shift-left: w233 -> [w248]
          shift-right: [w241] -> _
          shift-left: w229 -> [w242]
          stop <- w254 stop-if-true
          # ">wait cntr>"
          # "Step through\ncontrol event handle"
          # ">Dev refs>"
          # ">axis param>"
          # "Use -1 index for command array\nif need to quit loop prematuraly.\n-1 will go to default case \"End\""
          # ">loop cntr>"
          # ">prgm cntr>"
          n105 = case shown="True" "Step" {
            tunnel: w248 -> [w268 w269]
            tunnel: [w268 w269] -> w247
            frame False {
            }
            frame True {
              n106 = while {
                stop <- w270 stop-if-true
                n107 = event shown="[1] \"Next\": Value Change" {
                  selector: _ -> [_ _]
                  dyn-events: _ -> [_ _]
                  timeout: 100 -> [_ _]
                  tunnel: [_ "Next"] -> w270
                  event Timeout {
                    n108 = event-data() -> ()  [unwired: 1 in, 3 out]
                  }
                  event "Next": Value Change {
                    n109 = event-data() -> ()  [unwired: 1 in, 3 out]
                  }
                }
              }
            }
          }
          n110 = Index Array(array=w239, index=w240) -> (element=w238:T7)
          "Next command" <- w238
          n111 = Unbundle By Name(w238) -> ("Commands"=w243:T8, "Parameter1"=w267:dbl, "Parameter2"=w263:dbl, "Parameter3"=w250:dbl)  [unwired: 1 out]
          n112 = local read "Simulate Laser"() -> (w237:bool)
          n113 = Increment(x=w240) -> (x+1=w262:i32)
          n114 = case shown="\"X Move Abs\"" w243 {
            tunnel: w267 -> [_ _ _ w325 w347 w368 w388 _ w423 w459 w491 w512 _]
            tunnel: w266 -> [_ _ _ _ _ _ _ _ _ _ w492 _ _]
            tunnel: w265 -> [w287 w300 w313 w334 w356 w377 w397 w407 w429 w465 w490 w520 w527]
            tunnel: [w288 w301 w314 w335 w357 w378 w398 w406 w428 w464 w486 w521 w526] -> w264
            tunnel: w263 -> [_ _ _ w324 w346 w367 w387 _ _ _ w489 _ _]
            tunnel: w262 -> [w288 w301 w314 w335 w357 w378 w398 w406 w428 w464 w488 w523 w526]
            tunnel: [w287 w300 w313 w334 w356 w377 w397 w407 w429 w465 w482 w520 w527] -> w261
            tunnel: [w273 w290 w302 w317 w339 w359 w379 _ w409 w445 _ w493 TRUE] -> w257
            tunnel: w247 -> [w286 w299 w312 w332 w354 w375 w395 w400 w426 w462 w480 w513 w524]
            tunnel: w246 -> [w284 w296 w309 w328 w350 w371 w391 w401 w427 w463 _ w519 _]
            tunnel: w253 -> [w281 w297 w310 w326 w348 w369 w389 _ _ _ _ w517 _]
            tunnel: [w274 w289 w304 w315 w337 w361 w381 w400 w410 w446 w480 w495 w524] -> w251
            tunnel: [w275 w291 w303 w318 w340 w360 w380 _ w418 w455 _ w494 _] -> w252
            tunnel: w250 -> [_ _ _ w323 w345 w366 w386 _ _ _ _ _ _]
            tunnel: w242 -> [_ _ _ _ _ _ _ _ _ _ _ w506 _]
            tunnel: [_ _ _ _ _ _ _ _ _ _ _ w503 _] -> w241
            tunnel: w237 -> [_ _ _ _ _ _ _ _ w408 w444 _ _ _]
            tunnel: "Accel Ena" -> [_ _ _ w316 w338 _ _ _ _ _ _ _ _]
            frame "Home All" {
              n115 = Unbundle By Name(w284) -> ("Zaber Com"=w279:refnum<visa-resource-name>)
              n116 = Unbundle By Name(w281) -> ("Y"=w280:T3)
              n117 = Unbundle By Name(w281) -> ("X"=w283:T3)
              n118 = call "Zaber-home-v2.vi"("Lockstep?"=FALSE, "error in"=w286, "Zaber parameters"=w283, "Com Port"=w279) -> ("error out"=w282:errorcluster)  [unwired: 5 in, 2 out]
              n119 = call "Zaber-home-v2.vi"("Lockstep?"=TRUE, "error in"=w282, "Zaber parameters"=w280, "Com Port"=w279) -> ("error out"=w274:errorcluster)  [unwired: 5 in, 2 out]
              n120 = Unbundle By Name(w274) -> ("status"=w273:bool)
              n121 = Select(t="Zaber", s=w273, f="") -> (s? t:f=w275:string)
            }
            frame "X Home" {
              n122 = Unbundle By Name(w296) -> ("Zaber Com"=w294:refnum<visa-resource-name>)
              n123 = Unbundle By Name(w297) -> ("X"=w295:T3)
              n124 = call "Zaber-home-v2.vi"("Lockstep?"=FALSE, "error in"=w299, "Zaber parameters"=w295, "Com Port"=w294) -> ("error out"=w289:errorcluster)  [unwired: 5 in, 2 out]
              n125 = Unbundle By Name(w289) -> ("status"=w290:bool)
              n126 = Select(t="Zaber", s=w290, f="") -> (s? t:f=w291:string)
            }
            frame "Y Home" {
              n127 = Unbundle By Name(w309) -> ("Zaber Com"=w307:refnum<visa-resource-name>)
              n128 = Unbundle By Name(w310) -> ("Y"=w308:T3)
              n129 = call "Zaber-home-v2.vi"("Lockstep?"=TRUE, "error in"=w312, "Zaber parameters"=w308, "Com Port"=w307) -> ("error out"=w304:errorcluster)  [unwired: 5 in, 2 out]
              n130 = Unbundle By Name(w304) -> ("status"=w302:bool)
              n131 = Select(t="Zaber", s=w302, f="") -> (s? t:f=w303:string)
            }
            frame "X Move Rel" {
              w330 = TRUE  # Wait to complete
              w331 = FALSE  # Lockstep?
              n132 = local write "Accel Active"(w316) -> ()
              n133 = Bundle By Name(cluster=w326, "X.Move (units)"=w325, "X.Direction(-1,1)"=w324, "X.Speed (units/s)"=w323) -> (w322:T2)
              n134 = Unbundle By Name(w328) -> ("Zaber Com"=w327:refnum<visa-resource-name>)
              n135 = Unbundle By Name(w322) -> ("X"=w321:T3)
              n136 = call "Zaber-move-1-axis-v2.vi"("Lockstep?"=w331, "Wait to complete"=w330, "Movement Type"=enum16{"relative", "absolute"}."relative", "error in"=w332, "Zaber parameters"=w321, "Port In"=w327) -> ("error out"=w315:errorcluster)  [unwired: 3 in, 2 out]
              n137 = Unbundle By Name(w315) -> ("status"=w317:bool)
              n138 = flat-sequence {
                tunnel: w315 -> [_]
                frame #0 {
                  n139 = local write "Accel Active"(FALSE ("Accel Activ")) -> ()
                }
              }
              n140 = Select(t="Zaber", s=w317, f="") -> (s? t:f=w318:string)
              n141 = Wait (ms)(milliseconds to wait=u32 1) -> ()  [unwired: 1 out]
            }
            frame "X Move Abs" {
              w352 = TRUE  # Wait to complete
              w353 = FALSE  # Lockstep?
              n142 = local write "Accel Active"(w338) -> ()
              n143 = Bundle By Name(cluster=w348, "X.Move (units)"=w347, "X.Direction(-1,1)"=w346, "X.Speed (units/s)"=w345) -> (w344:T2)
              n144 = Unbundle By Name(w350) -> ("Zaber Com"=w349:refnum<visa-resource-name>)
              n145 = Unbundle By Name(w344) -> ("X"=w343:T3)
              n146 = call "Zaber-move-1-axis-v2.vi"("Lockstep?"=w353, "Wait to complete"=w352, "Movement Type"=enum16{"relative", "absolute"}."absolute", "error in"=w354, "Zaber parameters"=w343, "Port In"=w349) -> ("error out"=w337:errorcluster)  [unwired: 3 in, 2 out]
              n147 = Unbundle By Name(w337) -> ("status"=w339:bool)
              n148 = flat-sequence {
                tunnel: w337 -> [_]
                frame #0 {
                  n149 = local write "Accel Active"(FALSE ("Accel Activ")) -> ()
                }
              }
              n150 = Select(t="Zaber", s=w339, f="") -> (s? t:f=w340:string)
              n151 = Wait (ms)(milliseconds to wait=u32 1) -> ()  [unwired: 1 out]
            }
            frame "Y Move Rel" {
              w373 = TRUE  # Wait to complete
              w374 = TRUE  # Lockstep?
              n152 = Bundle By Name(cluster=w369, "Y.Move (units)"=w368, "Y.Direction(-1,1)"=w367, "Y.Speed (units/s)"=w366) -> (w365:T2)
              n153 = Unbundle By Name(w371) -> ("Zaber Com"=w370:refnum<visa-resource-name>)
              n154 = Unbundle By Name(w365) -> ("Y"=w364:T3)
              n155 = call "Zaber-move-1-axis-v2.vi"("Lockstep?"=w374, "Wait to complete"=w373, "Movement Type"=enum16{"relative", "absolute"}."relative", "error in"=w375, "Zaber parameters"=w364, "Port In"=w370) -> ("error out"=w361:errorcluster)  [unwired: 3 in, 2 out]
              n156 = Unbundle By Name(w361) -> ("status"=w359:bool)
              n157 = Select(t="Zaber", s=w359, f="") -> (s? t:f=w360:string)
              n158 = Wait (ms)(milliseconds to wait=u32 100) -> ()  [unwired: 1 out]
            }
            frame "Y Move Abs" {
              w393 = TRUE  # Wait to complete
              w394 = TRUE  # Lockstep?
              n159 = Bundle By Name(cluster=w389, "Y.Move (units)"=w388, "Y.Direction(-1,1)"=w387, "Y.Speed (units/s)"=w386) -> (w385:T2)
              n160 = Unbundle By Name(w391) -> ("Zaber Com"=w390:refnum<visa-resource-name>)
              n161 = Unbundle By Name(w385) -> ("Y"=w384:T3)
              n162 = call "Zaber-move-1-axis-v2.vi"("Lockstep?"=w394, "Wait to complete"=w393, "Movement Type"=enum16{"relative", "absolute"}."absolute", "error in"=w395, "Zaber parameters"=w384, "Port In"=w390) -> ("error out"=w381:errorcluster)  [unwired: 3 in, 2 out]
              n163 = Unbundle By Name(w381) -> ("status"=w379:bool)
              n164 = Select(t="Zaber", s=w379, f="") -> (s? t:f=w380:string)
              n165 = Wait (ms)(milliseconds to wait=u32 100) -> ()  [unwired: 1 out]
            }
            frame "Reset Intlk Timer" {
              n166 = Unbundle By Name(w401) -> ("MCU Com"=w399:refnum<visa-resource-name>)
              n167 = call "AR-Interlock-monitor-v2.vi"("Action"=AR-Interlock-monitor-comands."Clear Data", "error in"=w400, "Inlk Com"=w399) -> ("error out"=w404:errorcluster)  [unwired: 4 in, 4 out]
              n168 = call "AR-Interlock-monitor-v2.vi"("Action"=AR-Interlock-monitor-comands."Request", "error in"=w404, "Inlk Com"=w399) -> ("error out"=w405:errorcluster)  [unwired: 4 in, 4 out]
              n169 = call <vilib>:"Clear Errors.vi"("error in (no error)"=w405) -> ()  [unwired: 5 in, 2 out]
            }
            frame "Laser Sys ON" {
              n170 = Equal?(x=w423, y=1.0) -> (x = y?=w414:bool)
              n171 = Unbundle By Name(w427) -> ("LaserSysRef Out"=w425:refnum<k24>, "LaserControl Ref Out"=w424:refnum<k24>)
              n172 = Select(t=nLight-wait-states."Wait SysON" ("Action"), s=w414, f=nLight-wait-states."Wait SysOFF" ("Action")) -> (s? t:f=w411:T21)
              n173 = call "nLight-SystemON-ENA.vi"("ENA"=FALSE, "SysON"=w414, "Simulate (F)"=w408, "error in"=w426, "LaserControl Ref"=w424, "LaserSysRef"=w425) -> ("error out"=w417:errorcluster, "LaserControl Ref Out"=w416:refnum<k24>, "LaserSysRef Out"=w415:refnum<k24>)  [unwired: 3 in]
              n174 = disable-structure shown="Enabled" {
                disable-tunnel: w417 -> [w439 w442]
                disable-tunnel: w416 -> [w438 _]
                disable-tunnel: w415 -> [w437 _]
                disable-tunnel: w411 -> [w436 _]
                disable-tunnel: [w432 w441] -> w410
                disable-tunnel: [w431 FALSE] -> w409
                disable-tunnel: w408 -> [w430 _]
                frame Disabled {
                  n175 = call "nLight-Wait-for-Status.vi"("Timeout (s)"=5.0, "Action"=w436, "error in"=w439, "Simulate (F)"=w430, "LaserControl Ref"=w438, "LaserSysRef"=w437) -> ("error out"=w432:errorcluster, "Error"=w434:bool, "Fault"=w433:bool)  [unwired: 3 out]
                  n176 = Compound Arithmetic op=OR(w433, w434, w432) -> (w431:bool)
                }
                frame Enabled {
                  n177 = call "Sys on"("error in (no error)"=w442, "Delay Time (s)"=5.0) -> ("error out"=w441:errorcluster)  [unwired: 9 in]
                }
              }
              n178 = Select(t="Laser", s=w409, f="") -> (s? t:f=w418:string)
            }
            frame "Laser ENA" {
              n179 = Equal?(x=w459, y=1.0) -> (x = y?=w448:bool)
              n180 = Unbundle By Name(w463) -> ("LaserSysRef Out"=w461:refnum<k24>, "LaserControl Ref Out"=w460:refnum<k24>)
              n181 = Select(t=nLight-wait-states."Wait ENA" ("Action"), s=w448, f=nLight-wait-states."Wait DIS" ("Action")) -> (s? t:f=w449:T21)
              n182 = call "nLight-SystemON-ENA.vi"("ENA"=w448, "SysON"=TRUE, "Simulate (F)"=w444, "error in"=w462, "LaserControl Ref"=w460, "LaserSysRef"=w461) -> ("error out"=w454:errorcluster, "LaserControl Ref Out"=w453:refnum<k24>, "LaserSysRef Out"=w452:refnum<k24>)  [unwired: 3 in]
              n183 = disable-structure shown="Enabled" {
                disable-tunnel: w454 -> [w475 w478]
                disable-tunnel: w453 -> [w474 _]
                disable-tunnel: w452 -> [w473 _]
                disable-tunnel: w449 -> [w472 _]
                disable-tunnel: [w468 w477] -> w446
                disable-tunnel: [w467 FALSE] -> w445
                disable-tunnel: w444 -> [w466 _]
                frame Disabled {
                  n184 = call "nLight-Wait-for-Status.vi"("Timeout (s)"=5.0, "Action"=w472, "error in"=w475, "Simulate (F)"=w466, "LaserControl Ref"=w474, "LaserSysRef"=w473) -> ("error out"=w468:errorcluster, "Error"=w470:bool, "Fault"=w469:bool)  [unwired: 3 out]
                  n185 = Compound Arithmetic op=OR(w469, w470, w468) -> (w467:bool)
                }
                frame Enabled {
                  n186 = call "ENA delay"("error in (no error)"=w478, "Delay Time (s)"=5.0) -> ("error out"=w477:errorcluster)  [unwired: 9 in]
                }
              }
              n187 = Select(t="Laser", s=w445, f="") -> (s? t:f=w455:string)
            }
            frame "Repeat" {
              n188 = Search 1D Array(1D array=w492, element=w491) -> (index of element=w487:i32)  [unwired: 1 in]
              n189 = Increment(x=w490) -> (x+1=w484:i32)
              n190 = Less Or Equal?(x=w489, y=w484) -> (x <= y?=w485:bool)
              n191 = Select(t=w488, s=w485, f=w487) -> (s? t:f=w486:i32)
              n192 = Select(t=0, s=w485, f=w484) -> (s? t:f=w482:i32)
              n193 = Wait (ms)(milliseconds to wait=u32 100) -> ()  [unwired: 1 out]
            }
            frame "Wait" {
              # "Wait is implemented by looping through the same Wait state\n(doesn't increment the \"prgm cntr\" untill Timer expires."
              # "Properly reset timer\nthe first time it enters \nthe wait state"
              # "Update pos/speed\ngraph"
              n194 = Unbundle By Name(w517) -> ("X.Microstep Size"=w516:dbl, "X.Device (dev axis)"=w515:string, "X.Units"=w514:T9)
              n195 = Unbundle By Name(w519) -> ("Zaber Com"=w518:refnum<visa-resource-name>)
              n196 = call <instrlib>:"Read Current Position.vi"("Units (0: microsteps)"=w514, "error in (no error)"=w513, "Device and Axis"=w515, "Microstep Size (0)"=w516, "VISA resource name"=w518) -> ("error out"=w495:errorcluster, "Position"=w502:dbl)  [unwired: 4 in, 1 out]
              n197 = local write "X Position"(w502) -> ()
              n198 = Unbundle By Name(w495) -> ("status"=w493:bool)
              n199 = Equal To 0?(x=w506) -> (x = 0?=w511:bool)
              n200 = Select(t=enum16{"Reset", "Start"}."Reset" ("Action"), s=w511, f=enum16{"Reset", "Start"}."Start") -> (s? t:f=w509:enum16{"Reset", "Start"})
              n201 = Increment(x=w506) -> (x+1=w505:i32)
              n202 = Select(t="Zaber", s=w493, f="") -> (s? t:f=w494:string)
              n203 = call "Elapsed-Timer.vi"("Action"=w509, "Target (mS)"=w512) -> ("Time Elapsed"=w507:bool, "Loop time (ms)"=w501:u32)  [unwired: 7 in, 1 out]
              n204 = call "AR-Build-Axis-position-speed-graph.vi"("Select"="Select", "Action"=enum16{"Init", "WR", "RD"}."WR", "Loop time"=w501, "X Pos"=w502) -> ("Pos/Speed"=→"X Axis Pos/Speed":cluster{u32[], dbl[]})  [unwired: 7 in]
              n205 = Select(t=0, s=w507, f=w505) -> (s? t:f=w503:i32)
              n206 = Decrement(x=w523) -> (x-1=w522:i32)
              n207 = Select(t=w523, s=w507, f=w522) -> (s? t:f=w521:i32)
            }
            frame "End", Default {
            }
          }
          n208 = call "Stop-FGV.vi"("Action (RD)"=enum16{"Init", "WR", "RD"}."RD") -> ("Out"=w258:bool)  [unwired: 9 in, 1 out]
          n209 = Compound Arithmetic op=OR(w257, w258, "Stop") -> (w254:bool)
          n210 = Not(x=w254) -> (.not. x?=w256:bool)
          n211 = local read "msg-var"() -> (w245:T1)
          n212 = Bundle By Name(cluster=w245, "Run Rcp"=w256, "Rcp Stopped"=w254, "Err Device"=w252) -> (w244:T1)
          n213 = call "AR-msg-vars-FGV.vi"("Action"=enum16{"Init", "WR", "RD"}."WR", "msg-var in"=w244) -> ()  [unwired: 8 in, 2 out]
        }
        n214 = property on="Stop" class="Bool"("DisabledEnum"=T20."Enabled" ("Disabled")) -> ()  [unwired: 2 in, 2 out]
      }
    }
    n215 = call "Stop-FGV.vi"("Action (RD)"=enum16{"Init", "WR", "RD"}."RD") -> ("Out"=w225:bool)  [unwired: 9 in, 1 out]
  }
  n216 = while {
    shift-right: [w543] -> w10
    shift-left: w3 -> [w544]
    shift-right: [w541] -> _
    shift-left: "Init" ("Action") -> [w538]
    shift-right: [w536] -> _
    shift-left: T15 {"Zaber Com"="", "MCU Com"="", "LaserSysRef Out"=refnum, "LaserControl Ref Out"=refnum} ("Instr Refs") -> [w537]
    shift-right: [w532] -> _
    shift-left: T2 {"X"={"Device (dev axis)"="1 3", "Lockstep Group (1)"=1, "Units"=enum."millimeters", "Microstep Size"=4.21875, "Move (units)"=0.0, "Direction(-1,1)"=1, "Speed (units/s)"=1500.0}, "Y"={"Device (dev axis)"="1", "Lockstep Group (1)"=1, "Units"=enum."millimeters", "Microstep Size"=0.496094, "Move (units)"=0.0, "Direction(-1,1)"=1, "Speed (units/s)"=45.0}} ("Axis params") -> [w535]
    tunnel: w22 -> [w534]
    stop <- w539 stop-if-true
    # ">Dev refs>"
    # ">axis param>"
    n217 = local read "Simulate Laser"() -> (w530:bool)
    n218 = Wait (ms)(milliseconds to wait=u32 10) -> ()  [unwired: 1 out]
    n219 = case shown="\"Init\", Default" w538 {
      selector: w538 -> [_ _ w635 _ w676 _ w867]
      tunnel: [w556 w609 w634 w657 w677 w833 w854] -> w543
      tunnel: w544 -> [w559 w628 w645 w655 w678 w830 w862]
      tunnel: [w552 w605 w631 w660 w679 "Commands" ("Action") w867] -> w540
      tunnel: [_ _ _ _ _ _ w865] -> w539
      tunnel: w537 -> [w558 w619 w647 w659 w673 w824 w858]
      tunnel: [w557 w619 w647 w659 w673 w824 w858] -> w536
      tunnel: ["Axis params" w627 w648 w658 w674 w832 w864] -> w532
      tunnel: w535 -> [_ w627 w648 w658 w675 w832 w864]
      tunnel: w534 -> [w551 _ _ _ _ _ _]
      tunnel: "Recipe (csv)" -> [w555 _ _ _ w672 _ _]
      tunnel: w530 -> [w546 w616 _ _ w671 w821 w851]
      frame "Init", Default {
        n220 = event shown="[1] Timeout" {
          selector: _ -> [_ _]
          dyn-events: _ -> [_ _]
          timeout: 100 -> [_ _]
          tunnel: w559 -> [w568 w593]
          tunnel: [w589 w600] -> w548
          tunnel: [w569 w593] -> w556
          tunnel: w555 -> [w566 _]
          tunnel: "Com ports" -> [w588 w602]
          tunnel: [w583 w595] -> w552
          tunnel: w551 -> [w582 _]
          tunnel: [w573 w601] -> w547
          tunnel: [w562 _] -> w550
          tunnel: [w563 _] -> w549
          tunnel: w546 -> [w561 _]
          event "Init": Value Change {
            # "Some housekeeping"
            n221 = event-data() -> ()  [unwired: 1 in, 6 out]
            n222 = Unbundle By Name(w588) -> ("Zaber Com"=w589:refnum<visa-resource-name>, "Laser IP"=w581:string, "MCU Com"=w573:refnum<visa-resource-name>)
            n223 = call "Read-exec-script.vi"("error in"=w568, "file (use dialog)"=w566) -> ("error out"=w567:errorcluster, "Commands"=w565:T7[])  [unwired: 7 in, 1 out]
            n224 = local write "Script"(w565) -> ()
            n225 = for {
              tunnel: w582 -> [w592] mode=indexing
              n226 = property class="Page"(reference=w592, "PageEnb"=T17."Page Enabled" ("Page Enabled State")) -> ()  [unwired: 1 in, 2 out]
            }
            n227 = call <vilib>:"Clear Errors.vi"("error in (no error)"=w567) -> ("error out"=w580:errorcluster)  [unwired: 5 in, 1 out]
            n228 = call "nLight-Connect-Clear.vi"("Simulate?"=w561, "error in"=w580, "targetIpAddress"=w581) -> ("error out"=w564:errorcluster, "IsConnected"=w574:bool, "LaserControl Ref Out"=w563:refnum<k24>, "LaserSysRef Out"=w562:refnum<k24>)  [unwired: 5 in]
            "Laser OK" <- w574
            n229 = call "AR-Interlock-monitor-v2.vi"("Action"=AR-Interlock-monitor-comands."Init", "error in"=w580, "Inlk Com"=w573) -> ("error out"=w576:errorcluster)  [unwired: 4 in, 4 out]
            n230 = call "Zaber-multi-init.vi"("Log @"="At init stage", "error in (no error)"=w580, "Port #"=w589) -> ("error IO"=w560:errorcluster, "Port OK"=w587:bool)  [unwired: 3 in, 4 out]
            "Zaber OK" <- w587
            n231 = property on="Init" class="Bool"("DisabledEnum"=T20."Disabled" ("Disabled")) -> (error out=w571:errorcluster)  [unwired: 2 in, 1 out]
            n232 = property on="Quit" class="Bool (strict)"(error in=w571, "DisabledEnum"=T20."Enabled" ("Disabled")) -> ()  [unwired: 1 in, 2 out]
            n233 = Select(t=FALSE, s=w576, f=TRUE) -> (s? t:f=w575:bool)
            "MCU INLK" <- w575
            n234 = Compound Arithmetic op=AND(w574, w575, w587) -> (w586:bool)
            n235 = Select(t="Enable Mon Loop" ("f"), s=w586, f="Quit") -> (s? t:f=w583:string)
            n236 = Merge Errors(w564, w576, w560) -> (w569:errorcluster)
          }
          event Timeout {
            w599 = T20."Disabled and Grayed Out" ("Disabled")
            w598 = FALSE
            n237 = event-data() -> ()  [unwired: 1 in, 1 out]
            n238 = Unbundle By Name(w602) -> ("MCU Com"=w601:refnum<visa-resource-name>, "Zaber Com"=w600:refnum<visa-resource-name>)
            n239 = local write "Mode RDY"(w598) -> ()
            n240 = property on="MCU INLK" class="Bool"("Value"=w598) -> ()  [unwired: 2 in, 2 out]
            n241 = property on="Zaber OK" class="Bool"("Value"=w598) -> ()  [unwired: 2 in, 2 out]
            n242 = property on="Quit" class="Bool (strict)"("DisabledEnum"=T20."Enabled" ("Disabled")) -> ()  [unwired: 2 in, 2 out]
            n243 = property on="Laser OK" class="Bool"("Value"=w598) -> ()  [unwired: 2 in, 2 out]
            n244 = property on="Init" class="Bool"("DisabledEnum"=T20."Enabled" ("Disabled")) -> ()  [unwired: 2 in, 2 out]
            n245 = property on="ENA" class="Bool (strict)"("DisabledEnum"=w599) -> ()  [unwired: 2 in, 2 out]
            n246 = property on="Next" class="Bool"("DisabledEnum"=w599) -> ()  [unwired: 2 in, 2 out]
            n247 = property on="EMIT!" class="Bool (strict)"("DisabledEnum"=w599) -> ()  [unwired: 2 in, 2 out]
            n248 = local read "Quit"() -> (w594:bool)
            n249 = Select(t="Quit", s=w594, f="Init") -> (s? t:f=w595:string)
          }
        }
        n250 = Bundle By Name(cluster=w558, "MCU Com"=w547, "Zaber Com"=w548, "LaserSysRef Out"=w550, "LaserControl Ref Out"=w549) -> (w557:T15)
      }
      frame "Enable Mon Loop" {
        w614 = 1 items=["HW", "API", "CLI", "INET, CONTROL_INT_MASK"] ("ControllingInterface")
        n251 = call "Time Delay2"("error in (no error)"=w628, "Delay Time (s)"=0.5) -> ("error out"=w622:errorcluster)  [unwired: 9 in]
        n252 = local read "msg-var"() -> (w626:T1)
        n253 = Bundle By Name(cluster=w626, "Run Axis Loop"=TRUE) -> (w625:T1)
        n254 = Unbundle By Name(w619) -> ("LaserSysRef Out"=w617:refnum<k24>, "LaserControl Ref Out"=w618:refnum<k24>)
        n255 = call "AR-msg-vars-FGV.vi"("Action"=enum16{"Init", "WR", "RD"}."WR", "error in"=w622, "msg-var in"=w625) -> ("error out"=w620:errorcluster)  [unwired: 7 in, 1 out]
        n256 = call "nLight-Check-Control-Interface.vi"("Simulate (F)"=w616, "error in"=w620, "LaserControl Ref"=w618, "LaserSysRef"=w617) -> ("error out"=w609:errorcluster, "ExternalGate"=w611:bool, "ControllingInterface"=w615:i32, "ProfileModeEnabled"=w613:bool)  [unwired: 2 in, 2 out]
        "Controll Interface" <- w615
        "External Gate" <- w611
        "Profile Mode" <- w613
        n257 = Not(x=w613) -> (.not. x?=w610:bool)
        n258 = Equal?(x=w614, y=w615) -> (x = y?=w612:bool)
        n259 = Compound Arithmetic op=AND(w612, w611, w610) -> (w608:bool)
        n260 = case shown="False" w608 {
          frame False {
            n261 = One Button Dialog(message="Laser must be configured as API(GUI) Control Interface with External Gate control.\n\nCheck the Laser configuration in nLight Application and try again.") -> ()  [unwired: 1 in, 1 out]
          }
          frame True {
          }
        }
        n262 = Select(t="Test MCU Flags" ("Action"), s=w608, f="Quit" ("Action")) -> (s? t:f=w605:string)
      }
      frame "Test MCU Flags" {
        # "Repeat if flags are not set correctly\nOnly 1 at a time"
        n263 = Unbundle By Name(w647) -> ("MCU Com"=w644:refnum<visa-resource-name>)
        n264 = call "AR-Interlock-monitor-v2.vi"("Action"=AR-Interlock-monitor-comands."Request", "error in"=w645, "Inlk Com"=w644) -> ("error out"=w634:errorcluster, "Intlk Data"=w642:T12)  [unwired: 4 in, 3 out]
        n265 = Unbundle By Name(w642) -> ("Chamber Ena"=w640:bool, "Profiler Ena"=w639:bool, "OPower Ena"=w638:bool)
        n266 = Bundle By Name(cluster=T6 {"Chamber Ena"=FALSE, "Profiler Ena"=FALSE, "OPower Ena"=FALSE} ("MCU Gating Flags"), "Chamber Ena"=w640, "Profiler Ena"=w639, "OPower Ena"=w638) -> (→"MCU Gating Flags":T6)
        n267 = Compound Arithmetic op=XOR(w640, w639, w638) -> (w636:bool)
        n268 = case shown="False" w636 {
          tunnel: [w649 TRUE ("T button?")] -> w633
          frame False {
            n269 = Two Button Dialog(message="MCU Gating Control\n\nOnly 1 flag must be enabled in order for the Laser Gate control to be active.\nSet the correct Flags and click OK.\n\nClicking on Quit will terminate the program.", 1:"Quit" ("F button name (\"Cancel\")")) -> (T button?=w649:bool)  [unwired: 1 in]
          }
          frame True {
          }
        }
        n270 = Select(t="Test Gating" ("Action"), s=w636, f=w635) -> (s? t:f=w632:string)
        n271 = Select(t=w632, s=w633, f="Quit") -> (s? t:f=w631:string)
      }
      frame "Test Gating" {
        n272 = call "Display Message to User"("error in (no error)"=w655) -> ("error out"=w654:errorcluster, "YES"=w653:bool)  [unwired: 9 in]
        n273 = case shown="True" w653 {
          tunnel: [w663 w668] -> w657
          tunnel: w654 -> [w663 w664]
          frame False {
          }
          frame True {
            n274 = local read "Com ports"() -> (w670:T5)
            n275 = call "AR-Check-Gating.vi"("error in"=w664, "Zaber parameters"="X Axis Initial Test Parameters", "Com ports"=w670) -> ("error out"=w668:errorcluster, "Timed Out"=→"Gating Timedout":bool, "Time Delta (mS)"=→"Delta Time (mS)":dbl, "X Pos Triggered"=→"X Position Triggered":dbl)  [unwired: 5 in]
          }
        }
        n276 = Select(t="Commands" ("Action"), s=TRUE, f="Quit" ("Action")) -> (s? t:f=w660:string)
      }
      frame "Commands" {
        n277 = event shown="[11] \"Quit\": Value Change" {
          selector: _ -> [_ _ _ _ _ _ _ _ _ _ _ _]
          dyn-events: _ -> [_ _ _ _ _ _ _ _ _ _ _ _]
          timeout: 100 -> [_ _ _ _ _ _ _ _ _ _ _ _]
          tunnel: [w694 w710 w722 w732 w747 w756 w770 w785 w803 w814 "Test Gating" ("Action") "Quit" ("Action")] -> w679
          tunnel: w678 -> [w698 w700 w714 w728 w743 w764 w777 w784 w791 w812 w816 w819]
          tunnel: [w698 w700 w713 w723 w738 w757 w771 w783 w789 w811 w816 w819] -> w677
          tunnel: w676 -> [w690 w710 w722 w732 w747 w756 w770 w785 w803 w814 _ _]
          tunnel: w675 -> [w688 w705 w716 w731 w746 w765 w778 w787 w805 w813 w817 w818]
          tunnel: [w686 w705 w715 w731 w746 w765 w778 w787 w805 w813 w817 w818] -> w674
          tunnel: w673 -> [_ _ w712 _ _ w763 w776 w786 w804 w809 _ _]
          tunnel: w672 -> [_ _ _ w730 w745 _ _ _ _ _ _ _]
          tunnel: w671 -> [_ _ _ _ _ w754 w767 w780 w793 w807 _ _]
          event Timeout {
            n278 = event-data() -> ()  [unwired: 1 in, 1 out]
            n279 = Bundle By Name(cluster=w688, "X.Units"="Select Units", "Y.Units"="Select Units", "X.Device (dev axis)"="X (dev axis)", "Y.Device (dev axis)"="Y (dev axis)", "X.Microstep Size"="X Microstep Size", "Y.Microstep Size"="Y Microstep Size") -> (w686:T2)
            n280 = call "AR-msg-vars-FGV.vi"("Action"=enum16{"Init", "WR", "RD"}."RD") -> ("msg-var"=w692:T1)  [unwired: 9 in, 1 out]
            "msg-var" <- w692
            n281 = Unbundle By Name(w692) -> ("Rcp Stopped"=w681:bool)
            n282 = case shown="False" w681 {
              frame False {
              }
              frame True {
                n283 = property on="Next" class="Bool"("DisabledEnum"=T20."Disabled and Grayed Out" ("Disabled")) -> ()  [unwired: 2 in, 2 out]
              }
            }
            n284 = Select(t="Safe", s=w681, f=w690) -> (s? t:f=w689:string)
            n285 = call "Stop-FGV.vi"("Action (RD)"=enum16{"Init", "WR", "RD"}."RD") -> ("Out"=w696:bool)  [unwired: 9 in, 1 out]
            n286 = Select(t="Quit", s=w696, f=w689) -> (s? t:f=w694:string)
          }
          event "Run script": Value Change {
            # "Ena Next Button\nwhen script started"
            n287 = event-data() -> ()  [unwired: 1 in, 1 out]
            n288 = local read "msg-var"() -> (w702:T1)
            n289 = Bundle By Name(cluster=w702, "Run Rcp"=TRUE, "Rcp Stopped"=FALSE ("Stop Rcp")) -> (w708:T1)
            n290 = call "AR-Build-Axis-position-speed-graph.vi"("Action"=enum16{"Init", "WR", "RD"}."Init", "error in (no error)"=w700) -> ()  [unwired: 9 in, 1 out]
            n291 = call "AR-msg-vars-FGV.vi"("Action"=enum16{"Init", "WR", "RD"}."WR", "msg-var in"=w708) -> ("error out"=w703:errorcluster)  [unwired: 8 in, 1 out]
            n292 = property on="Next" class="Bool"(error in=w703, "DisabledEnum"=T20."Enabled" ("Disabled")) -> ()  [unwired: 1 in, 2 out]
          }
          event "Zaber settings": Value Change {
            n293 = event-data() -> ()  [unwired: 1 in, 1 out]
            n294 = Unbundle By Name(w712) -> ("Zaber Com"=w711:refnum<visa-resource-name>)
            n295 = call "AR-Axis-update-parameters-GUI.vi"("error in"=w714, "Com"=w711) -> ("error out"=w713:errorcluster, "Axis"=→"Axis":string[], "Connected Devices"=→"Devices":string[], "Device Info"=→"Device Info":T10)  [unwired: 6 in]
            n296 = Bundle By Name(cluster=w716, "Y.Device (dev axis)"="1", "X.Device (dev axis)"="1 3") -> (w715:T2)
          }
          event "Load script": Value Change {
            n297 = event-data() -> ()  [unwired: 1 in, 1 out]
            n298 = Strip Path(path=w730) -> (stripped path=w729:path)  [unwired: 1 out]
            n299 = call "File Dialog"("start path"=w729, "error in"=w728) -> ("selected path"=w725:path, "cancelled"=w727:bool, "error out"=w726:errorcluster)  [unwired: 10 in, 1 out]
            n300 = case shown="False" w727 {
              tunnel: w726 -> [w736 w737]
              tunnel: w725 -> [w734 _]
              tunnel: [w735 w737] -> w724
              frame False {
                n301 = call "Read-exec-script.vi"("error in"=w736, "file (use dialog)"=w734) -> ("error out"=w735:errorcluster, "Commands"=w733:T7[])  [unwired: 7 in, 1 out]
                n302 = local write "Script"(w733) -> ()
              }
              frame True {
              }
            }
            n303 = call <vilib>:"Clear Errors.vi"("error in (no error)"=w724) -> ("error out"=w723:errorcluster)  [unwired: 5 in, 1 out]
          }
          event "Save script": Value Change {
            n304 = event-data() -> ()  [unwired: 1 in, 1 out]
            n305 = Strip Path(path=w745) -> (stripped path=w744:path)  [unwired: 1 out]
            n306 = call "File Dialog2"("start path"=w744, "error in"=w743) -> ("selected path"=w740:path, "cancelled"=w742:bool, "error out"=w741:errorcluster)  [unwired: 10 in, 1 out]
            n307 = case shown="False" w742 {
              tunnel: w741 -> [w751 w752]
              tunnel: w740 -> [w750 _]
              tunnel: [w748 w752] -> w739
              frame False {
                n308 = local read "Script"() -> (w749:T7[])
                n309 = call "Save-exec-script.vi"("error in"=w751, "Script array"=w749, "file (use dialog)"=w750) -> ("error out"=w748:errorcluster)  [unwired: 7 in, 1 out]
              }
              frame True {
              }
            }
            n310 = call <vilib>:"Clear Errors.vi"("error in (no error)"=w739) -> ("error out"=w738:errorcluster)  [unwired: 5 in, 1 out]
          }
          event "SysON": Value Change {
            w755 = T20."Disabled and Grayed Out" ("Disabled")
            w760 = FALSE  # ENA
            n311 = event-data() -> ("NewVal"=w753:bool)  [unwired: 1 in]
            n312 = Unbundle By Name(w763) -> ("LaserSysRef Out"=w762:refnum<k24>, "LaserControl Ref Out"=w761:refnum<k24>)
            n313 = call "nLight-SystemON-ENA.vi"("ENA"=w760, "SysON"=w753, "Simulate (F)"=w754, "error in"=w764, "LaserControl Ref"=w761, "LaserSysRef"=w762) -> ("error out"=w757:errorcluster)  [unwired: 3 in, 2 out]
            n314 = Select(t=T20."Enabled" ("Disabled"), s=w753, f=w755) -> (s? t:f=w758:T20)
            n315 = property on="ENA" class="Bool (strict)"("DisabledEnum"=w758) -> ()  [unwired: 2 in, 2 out]
            n316 = property on="EMIT!" class="Bool (strict)"("DisabledEnum"=w755) -> ()  [unwired: 2 in, 2 out]
          }
          event "ENA": Value Change {
            w769 = TRUE  # SysON
            n317 = event-data() -> ("NewVal"=w766:bool)  [unwired: 1 in]
            n318 = Unbundle By Name(w776) -> ("LaserSysRef Out"=w775:refnum<k24>, "LaserControl Ref Out"=w774:refnum<k24>)
            n319 = call "nLight-SystemON-ENA.vi"("ENA"=w766, "SysON"=w769, "Simulate (F)"=w767, "error in"=w777, "LaserControl Ref"=w774, "LaserSysRef"=w775) -> ("error out"=w771:errorcluster)  [unwired: 3 in, 2 out]
            n320 = Select(t=T20."Enabled" ("Disabled"), s=w766, f=T20."Disabled and Grayed Out" ("Disabled")) -> (s? t:f=w768:T20)
            n321 = property on="EMIT!" class="Bool (strict)"("DisabledEnum"=w768) -> ()  [unwired: 2 in, 2 out]
          }
          event "EMIT!": Value Change {
            n322 = event-data() -> ("NewVal"=w779:bool)  [unwired: 1 in]
            n323 = Unbundle By Name(w786) -> ("LaserSysRef Out"=w782:refnum<k24>, "LaserControl Ref Out"=w781:refnum<k24>)
            n324 = call "nLight-Emit.vi"("Emit!"=w779, "Simulate (F)"=w780, "error in"=w784, "LaserControl Ref"=w781, "LaserSysRef"=w782) -> ("error out"=w783:errorcluster)  [unwired: 4 in, 2 out]
          }
          event "Set Laser Params": Value Change {
            n325 = event-data() -> ()  [unwired: 1 in, 1 out]
            n326 = Unbundle By Name(w804) -> ("LaserSysRef Out"=w802:refnum<k24>, "LaserControl Ref Out"=w801:refnum<k24>)
            n327 = property on="Mode RDY" class="Bool (strict)"(error in=w791, "Value"=FALSE ("Mode RDY")) -> ()  [unwired: 1 in, 2 out]
            n328 = call "nLight-Set-Laser-Params.vi"("Simulate (F)"=w793, "Laser Params"="Laser Params", "error in"=w791, "LaserControl Ref"=w801, "LaserSysRef"=w802) -> ("error out"=w796:errorcluster, "Comanded Params"=w799:T13, "LaserControl Ref Out"=w794:refnum<k24>, "LaserSysRef Out"=w795:refnum<k24>)  [unwired: 3 in]
            n329 = Unbundle By Name(w799) -> ("Power(W)"=→"Laser Power (W)":dbl, "Duty(%)"=→"Laser Duty (%)":dbl)
            n330 = call "nLight-Beam-Profile-Mode-SubVI.vi"("Simulate (F)"=w793, "error in"=w796, "Beam-profile(0-6)"="Beam-profile(0-6)", "LaserControl Ref"=w794, "LaserSysRef"=w795) -> ("error out"=w789:errorcluster)  [unwired: 2 in, 4 out]
            n331 = property on="Mode RDY" class="Bool (strict)"(error in=w789, "Value"=TRUE ("Mode RDY")) -> ()  [unwired: 1 in, 2 out]
          }
          event "AIMING": Value Change {
            n332 = event-data() -> ("NewVal"=w810:bool)  [unwired: 1 in]
            n333 = Unbundle By Name(w809) -> ("LaserControl Ref Out"=w808:refnum<k24>)
            n334 = call "nLight-Aiming-Mode-SubVI.vi"("AimingLaserOn"=w810, "Simulate (F)"=w807, "error in"=w812, "LaserControl Ref"=w808) -> ("error out"=w811:errorcluster, "Aiming ON"=→"Aiming RDY":bool)  [unwired: 4 in, 2 out]
          }
          event "Re-test gating": Value Change {
            n335 = event-data() -> ()  [unwired: 1 in, 1 out]
          }
          event "Quit": Value Change {
            n336 = event-data() -> ()  [unwired: 1 in, 1 out]
          }
        }
      }
      frame "Safe" {
        # "The Script execution has been stopped by the user"
        n337 = call "AR-msg-vars-FGV.vi"("Action"=enum16{"Init", "WR", "RD"}."RD", "error in"=w830) -> ("error out"=w828:errorcluster, "msg-var"=w829:T1)  [unwired: 8 in]
        n338 = Unbundle By Name(w824) -> ("LaserSysRef Out"=w823:refnum<k24>, "LaserControl Ref Out"=w822:refnum<k24>)
        n339 = Unbundle By Name(w829) -> ("Err Device"=w827:string)
        n340 = case shown="\"Zaber\", Default" w827 {
          tunnel: w828 -> [w846 w847]
          tunnel: [w841 w847] -> w826
          tunnel: w823 -> [w845 _]
          tunnel: w822 -> [w844 _]
          tunnel: w821 -> [w839 _]
          frame "Zaber", Default {
            w843 = FALSE ("SysON")
            # "If Zaber Err OR no Err, do Lase Safe Routine"
            n341 = call "nLight-SystemON-ENA.vi"("ENA"=w843, "SysON"=w843, "Simulate (F)"=w839, "error in"=w846, "LaserControl Ref"=w844, "LaserSysRef"=w845) -> ("error out"=w842:errorcluster)  [unwired: 3 in, 2 out]
            n342 = call "Time Delay"("error in (no error)"=w842, "Delay Time (s)"=2.0) -> ("error out"=w841:errorcluster)  [unwired: 9 in]
          }
          frame "Laser" {
            # "If Laser Err show warning Msg here, no Laser Safe routine"
            n343 = One Button Dialog(message="Laser Error") -> ()  [unwired: 1 in, 1 out]
          }
        }
        n344 = local read "msg-var"() -> (w825:T1)
        n345 = Bundle By Name(cluster=w825, "Run Rcp"=FALSE, "Rcp Stopped"=FALSE) -> (w837:T1)
        n346 = call "AR-msg-vars-FGV.vi"("Action"=enum16{"Init", "WR", "RD"}."WR", "error in"=w826, "msg-var in"=w837) -> ("error out"=w833:errorcluster)  [unwired: 7 in, 1 out]
      }
      frame "Quit" {
        w865 = TRUE
        n347 = call "AR-msg-vars-FGV.vi"("Action"=enum16{"Init", "WR", "RD"}."RD", "error in"=w862) -> ("error out"=w850:errorcluster, "msg-var"=w861:T1)  [unwired: 8 in]
        n348 = Unbundle By Name(w861) -> ("Err Device"=w859:string)
        n349 = call "Time Delay3"("error in (no error)"=w850) -> ("error out"=w849:errorcluster)  [unwired: 10 in]
        n350 = case shown="\"Zaber\"" w859 {
          tunnel: w858 -> [w880 w888]
          tunnel: w864 -> [_ w887]
          tunnel: [w881 w886] -> w860
          tunnel: w849 -> [w882 w885]
          frame "Zaber" {
            # "Zabe err do nothing, Msg?"
            n351 = Unbundle By Name(w880) -> ("Zaber Com"=w879:refnum<visa-resource-name>)
            n352 = One Button Dialog(message="Zaber Error") -> ()  [unwired: 1 in, 1 out]
            n353 = call <instrlib>:"Close.vi"("error in (no error)"=w882, "VISA resource name"=w879) -> ("error out"=w881:errorcluster)  [unwired: 9 in]
          }
          frame "No Err", Default {
            n354 = Unbundle By Name(w888) -> ("Zaber Com"=w884:refnum<visa-resource-name>)
            n355 = Unbundle By Name(w887) -> ()  [unwired: 1 out]
            n356 = Unbundle By Name(w887) -> ()  [unwired: 1 out]
            n357 = call <instrlib>:"Close.vi"("error in (no error)"=w885, "VISA resource name"=w884) -> ("error out"=w886:errorcluster)  [unwired: 9 in]
          }
        }
        n358 = Unbundle By Name(w858) -> ("MCU Com"=w852:refnum<visa-resource-name>, "LaserSysRef Out"=w856:refnum<k24>, "LaserControl Ref Out"=w857:refnum<k24>)
        n359 = case shown="\"No Err\", Default" w859 {
          tunnel: w860 -> [w877 w878]
          tunnel: [w876 w878] -> w855
          tunnel: w857 -> [w874 _]
          tunnel: w856 -> [w875 _]
          tunnel: w851 -> [w869 _]
          frame "No Err", Default {
            w870 = FALSE ("SysON")
            # "Laser Uninit here"
            n360 = call <vilib>:"Clear Errors.vi"("error in (no error)"=w877) -> ("error out"=w873:errorcluster)  [unwired: 5 in, 1 out]
            n361 = call "nLight-SystemON-ENA.vi"("ENA"=w870, "SysON"=w870, "Simulate (F)"=w869, "error in"=w873, "LaserControl Ref"=w874, "LaserSysRef"=w875) -> ("error out"=w872:errorcluster, "LaserSysRef Out"=w871:refnum<k24>)  [unwired: 3 in, 1 out]
            n362 = call "nLight-Disconnect.vi"("Simulate (F)"=w869, "error in"=w872, "LaserSysRef"=w871) -> ("error out"=w876:errorcluster)  [unwired: 8 in]
          }
          frame "Laser" {
            # "Laser Err, do nothing. There was a msg at \"Safe\" case"
          }
        }
        n363 = disable-structure shown="Enabled" {
          frame Disabled {
            n364 = One Button Dialog(message="Disable Laser, Home Axis, Uninit All") -> ()  [unwired: 1 in, 1 out]
          }
          frame Enabled {
          }
        }
        n365 = call "AR-Interlock-monitor-v2.vi"("Action"=AR-Interlock-monitor-comands."Close", "error in"=w855, "Inlk Com"=w852) -> ("error out"=w854:errorcluster)  [unwired: 4 in, 4 out]
        n366 = call "Stop-FGV.vi"("Action (RD)"=enum16{"Init", "WR", "RD"}."WR", "Action"=w865) -> ()  [unwired: 8 in, 2 out]
      }
    }
    "Instr Refs" <- w536
    n367 = local write "Axis params"(w532) -> ()
    n368 = Select(t="Quit" ("Action"), s=w543, f=w540) -> (s? t:f=w541:string)
    "Action" <- w538
  }
  n369 = while {
    tunnel: w3 -> [_]
    stop <- w891 stop-if-true
    # "Acceleration logging"
    n370 = Wait (ms)(milliseconds to wait=u32 1) -> ()  [unwired: 1 out]
    n371 = local read "Accel Active"() -> (w889:bool)
    n372 = case shown="True" w889 {
      frame False {
      }
      frame True {
        n373 = call <vilib>:"Create File with Incrementing Suffix.vi"("file path"="Accel CSV File") -> ("error out"=w894:errorcluster, "actual path"=w893:path)  [unwired: 8 in, 1 out]
        n374 = call "py_accel.vi"("Time Target (s)"="Target Time (s)", "error in"=w894, "Accel CSV file"=w893, "COM"="Accel COM") -> ("File OK"=→"File OK":bool, "Com\nError"=→"Com\nError":bool)  [unwired: 6 in]
      }
    }
    n375 = call "Stop-FGV.vi"("Action (RD)"=enum16{"Init", "WR", "RD"}."RD") -> ("Out"=w891:bool)  [unwired: 9 in, 1 out]
  }
  n376 = call "Stop-FGV.vi"("Action (RD)"=enum16{"Init", "WR", "RD"}."WR", "error in"=w11, "Action"=TRUE) -> ("error out"=w8:errorcluster)  [unwired: 7 in, 1 out]
  n377 = call "Stop-FGV.vi"("Action (RD)"=enum16{"Init", "WR", "RD"}."WR", "error in"=w16, "Action"=TRUE) -> ("error out"=w9:errorcluster)  [unwired: 7 in, 1 out]
  n378 = Merge Errors(w10, w9, w8) -> (w6:errorcluster)
  n379 = call "AR-msg-vars-FGV.vi"("Action"=enum16{"Init", "WR", "RD"}."RD", "error in"=w6) -> ("error out"=→"error out":errorcluster, "msg-var"=→"msg-var at exit":T1)  [unwired: 8 in]
